vi "Main.vi"() -> ()   [LabVIEW 2020]
uses:
  Main/Main Refs.ctl
  Hardware/Tecan/Pump Config.ctl
  Main/Timing Specs.ctl
  Main/Vacuum Specs.ctl
  Main/Cartridges.ctl
  Main/Cartridge Status.ctl
  Main/Commands.ctl
  Lib/Time/Wells.ctl
  Lib/Time/Bottles.ctl
  Main/Process State.ctl
  Main/Vacuum Test.ctl
  Hardware/Tecan/Pump Control.ctl
  Main/Pump Port.ctl
  Hardware/Tecan/Velocity Units.ctl
  Main/Pump Script Step.ctl
  Main/Script Step.ctl
  Main/Drain Valve.ctl
  Main/Wash Step.ctl
  Main/Zaber Controls.ctl
  Main/Vacuum Output.ctl
  Hardware/DAQ Mngr.ctl
  Main/Process Mngr.ctl
  Main/Cartridge Mngr.ctl
  Main/Script Mngr Action.ctl
  Main/Script Mngr Script choice.ctl
  Main/Time elapsed.ctl
  Hardware/Denkovi Mngr.ctl
  Hardware/Valco Valve/Valco Valve Mngr Action.ctl
  Hardware/Tricon Mngr.ctl
  Hardware/Mot Stage Mngr.ctl
  Main/Config Mngr.ctl
  Hardware/Hardware Globals.vi
  Main/Main Globals.vi
  Lib/Utilities.lvlib
  Hardware/Zaber/Zaber A Series.lvlib
panel:
  in  "Config 2":T1={"Syringe size"=0, "Syringe address"=0, "# of ports"=0, "Init String"="Z0N1R", "Full Stroke (cnts)"=0, "Model"=enum."XC", "TW Position"=0.0, "Load Position"=0.0, "Bottom Position"=0.0, "Station ID"="", "Default Protocol"=path "", "Dry Time(s)"=0.0, "Python Version"="", "NFC SN Array"=["21121521200223", "21121521200186", "21121521200213", "52541737200062"], "Timing"={"Checking pres and leak"=0.0, "Priming input lines"=0.0, "Rinsing syringe"=0.0, "Filling well X w/ X"=0.0, "Drain well X"=0.0, "Clearing wells and lines"=0.0, "Draining wells"=0.0, "Rinsing all wells"=0.0, "Testing for leaks/clogs"=0.0, "Rinsing wells"=0.0}, "Pressure Specs"={"Pressure max"=0.0, "Pressure min"=0.0, "Decay delta"=0.0, "Pressure time"=0.0, "Conf. R"=0.0, "LeakRateMax"=0.0}}
  out "Progress":u8(slide) scale=0.0..100.0
  in  "Software Mode":bool=TRUE
  out "Version":string
  out "error out":errorcluster
  in  "Main References":T4
  in  "Tab Control":T5(tab)
  in  "Init Hardware":bool
  in  "Main Clean Cart":bool
  out "Zaber Found":bool caption="Motion"
  out "Relays Found":bool caption="Relays"
  out "NI DAQ Found":bool caption="DAQ"
  out "Current Protocol":string
  out "Date":string
  out "Station":string="Fixture 1"
  in  "Operator":string
  in  "Time Remaining":string
  in  "Start TW":bool
  in  "Cartridges":T6
  out "Pump Found":bool caption="Pump"
  out "Valco Found":bool caption="Valves"
  in  "Commands":T8={"Drain All Wells"=FALSE, "Rinse All Wells"=FALSE, "Prime"=FALSE, "Well #"=enum."Well 1", "Bottle #"=enum."Bottle 1", "Fill"=FALSE, "Run State"=FALSE, "State"=enum."Fill Wells", "Empty Lines"=FALSE, "Clean&Dry Cartridge"=FALSE, "Check for leaks"=FALSE, "Cart Test Array"=[], "Number of rinses"=0.0} {"Number of rinses" min=1.0 max=50.0 step=1.0}
  in  "Protocol Save":bool
  in  "Protocol Load":bool
  out "Wash Setup File Path":path
  in  "Protocol Clear":bool
  in  "Wash Array":T13[](array[typedef]) {"# of Rinses" max=10}
  in  "Manual Subtab":T14(tab)
  in  "Fit Pnts":dbl
  in  "AutoLock":bool=TRUE
  in  "Zaber Save Bottom Pos":bool
  in  "Zaber Save Load Pos":bool
  in  "Zaber Save TW Pos":bool
  in  "Zaber Bottom_pos":bool
  in  "Zaber Load_pos":bool
  in  "Zaber TW_pos":bool
  in  "Man Cart Read":T15={"Cart1"=TRUE, "Cart2"=TRUE, "Cart3"=TRUE, "Cart4"=TRUE, "Cart 1 SN"="", "Cart 2 SN"="", "Cart 3 SN"="", "Cart 4 SN"=""}
  out "Cart Sense Cluster":T16
  in  "Man Cart Control":T16={"Cart1"=TRUE, "Cart2"=TRUE, "Cart3"=TRUE, "Cart4"=TRUE}
  in  "Man Pres Control":T17={"Vial1"=TRUE, "Vial2"=TRUE, "Vial3"=TRUE, "Vial4"=TRUE, "Vent"=TRUE, "Pressure"=TRUE, "Pinch Valve"=FALSE}
  in  "Man Valco":enum32{"Port1", "Port2", "Port3", "Port4"}(radio)
  in  "Syringe Pump":T18={"Syringe Pos"=0, "Rate"=0.0, "Volume"=0.0, "Valve"=enum."Bottle 1", "Action"=enum."Withdraw", "Move Type"=enum."Rel", "Init"=TRUE, "Empty Syr."=TRUE, "Full Fill"=TRUE, "Units"=enum."ul/s"} {"Syringe Pos" scale=0.0..2500.0}
  in  "Pump Cmd":string
  out "Pump Response":string
  in  "Send Cmd":bool
  in  "Man Peristaltic Ctrl":bool
  out "Pressure Level":cluster{"Time":dbl[], "Value":dbl[]}[](graph)
  in  "Motor Cluster":T21 {"Mot Rel Dist" min=0.0 max=400000.0; "Mot Abs Dist" format="%#.1f"; "Position(mm)" format="%.2f"}
  out "Data Array":T22[](array[typedef])
  in  "Man Script Step":u16
  out "Man Script Path":path
  in  "Man Script Run":bool
  in  "Manual Script Array":T23[](array[typedef])
  in  "Man Script Load":bool
  in  "Man Script Save":bool
  in  "Man Script Clear":bool
  in  "Pump Script Array":T25[](array[typedef])
  in  "Pump Save Script":bool
  in  "Pump Load Script":bool
  in  "Pump Script File":path
  in  "Pump Clear Script":bool
  in  "Pump Start Script":bool
  out "Reports":path
  out "Python Folder":path
  out "Data Folder":path
  out "Root path":path
  out "Config Folder":path
  out "Scripts Folder":path
  out "Logs Folder":path
  in  "Save Config":bool
  in  "Config":T1={"Syringe size"=0, "Syringe address"=0, "# of ports"=0, "Init String"="Z0N1R", "Full Stroke (cnts)"=0, "Model"=enum."XC", "TW Position"=0.0, "Load Position"=0.0, "Bottom Position"=0.0, "Station ID"="", "Default Protocol"=path "", "Dry Time(s)"=0.0, "Python Version"="", "NFC SN Array"=["21121521200223", "21121521200186", "21121521200213", "52541737200062"], "Timing"={"Checking pres and leak"=0.0, "Priming input lines"=0.0, "Rinsing syringe"=0.0, "Filling well X w/ X"=0.0, "Drain well X"=0.0, "Clearing wells and lines"=0.0, "Draining wells"=0.0, "Rinsing all wells"=0.0, "Testing for leaks/clogs"=0.0, "Rinsing wells"=0.0}, "Pressure Specs"={"Pressure max"=0.0, "Pressure min"=0.0, "Decay delta"=0.0, "Pressure time"=0.0, "Conf. R"=0.0, "LeakRateMax"=0.0}}
  out "Protocols Folder":path
  out "Run Time System?":bool
  out "Error":string
  out "Status":string
  # "Tecan Pump"
  # "Pressure"
  # "General"
  # "Timing"
  # "Protocol"
  # "Zaber"
  # "NFC Reader 1"
  # "NFC  Reader 2"
  # "NFC Reader 3"
  # "NFC Reader 4"
  # "Tecan Pump"
  # "Pressure"
  # "General"
  # "Timing"
  # "Protocol"
  # "Zaber"
  # "NFC Reader 1"
  # "NFC  Reader 2"
  # "NFC Reader 3"
  # "NFC Reader 4"
  # "System"
  # "Cartridge Utitlies"
  # "Wells"
  # "times"
  # "from"
  # "State Machine"
  # "System"
  # "Cartridge Utitlies"
  # "Wells"
  # "times"
  # "from"
  # "State Machine"
  # "Wash Protocol"
  # "Tecan Syringe Pump"
  # "Motion"
  # "Cartridges"
  # "Pressure"
  # "Tecan Serial Communication"
  # "Waste"
  # "Step"
  # "Volume"
  # "Rate"
  # "Valco"
  # "Peri"
  # "Pressure"
  # "Move Abs"
  # "Delay(s)"
  # "Tecan Pump"
  # "Pressure"
  # "General"
  # "Timing"
  # "Protocol"
  # "Zaber"
  # "NFC Reader 1"
  # "NFC  Reader 2"
  # "NFC Reader 3"
  # "NFC Reader 4"
  # "Software created by:\nYuri Kouchnir"
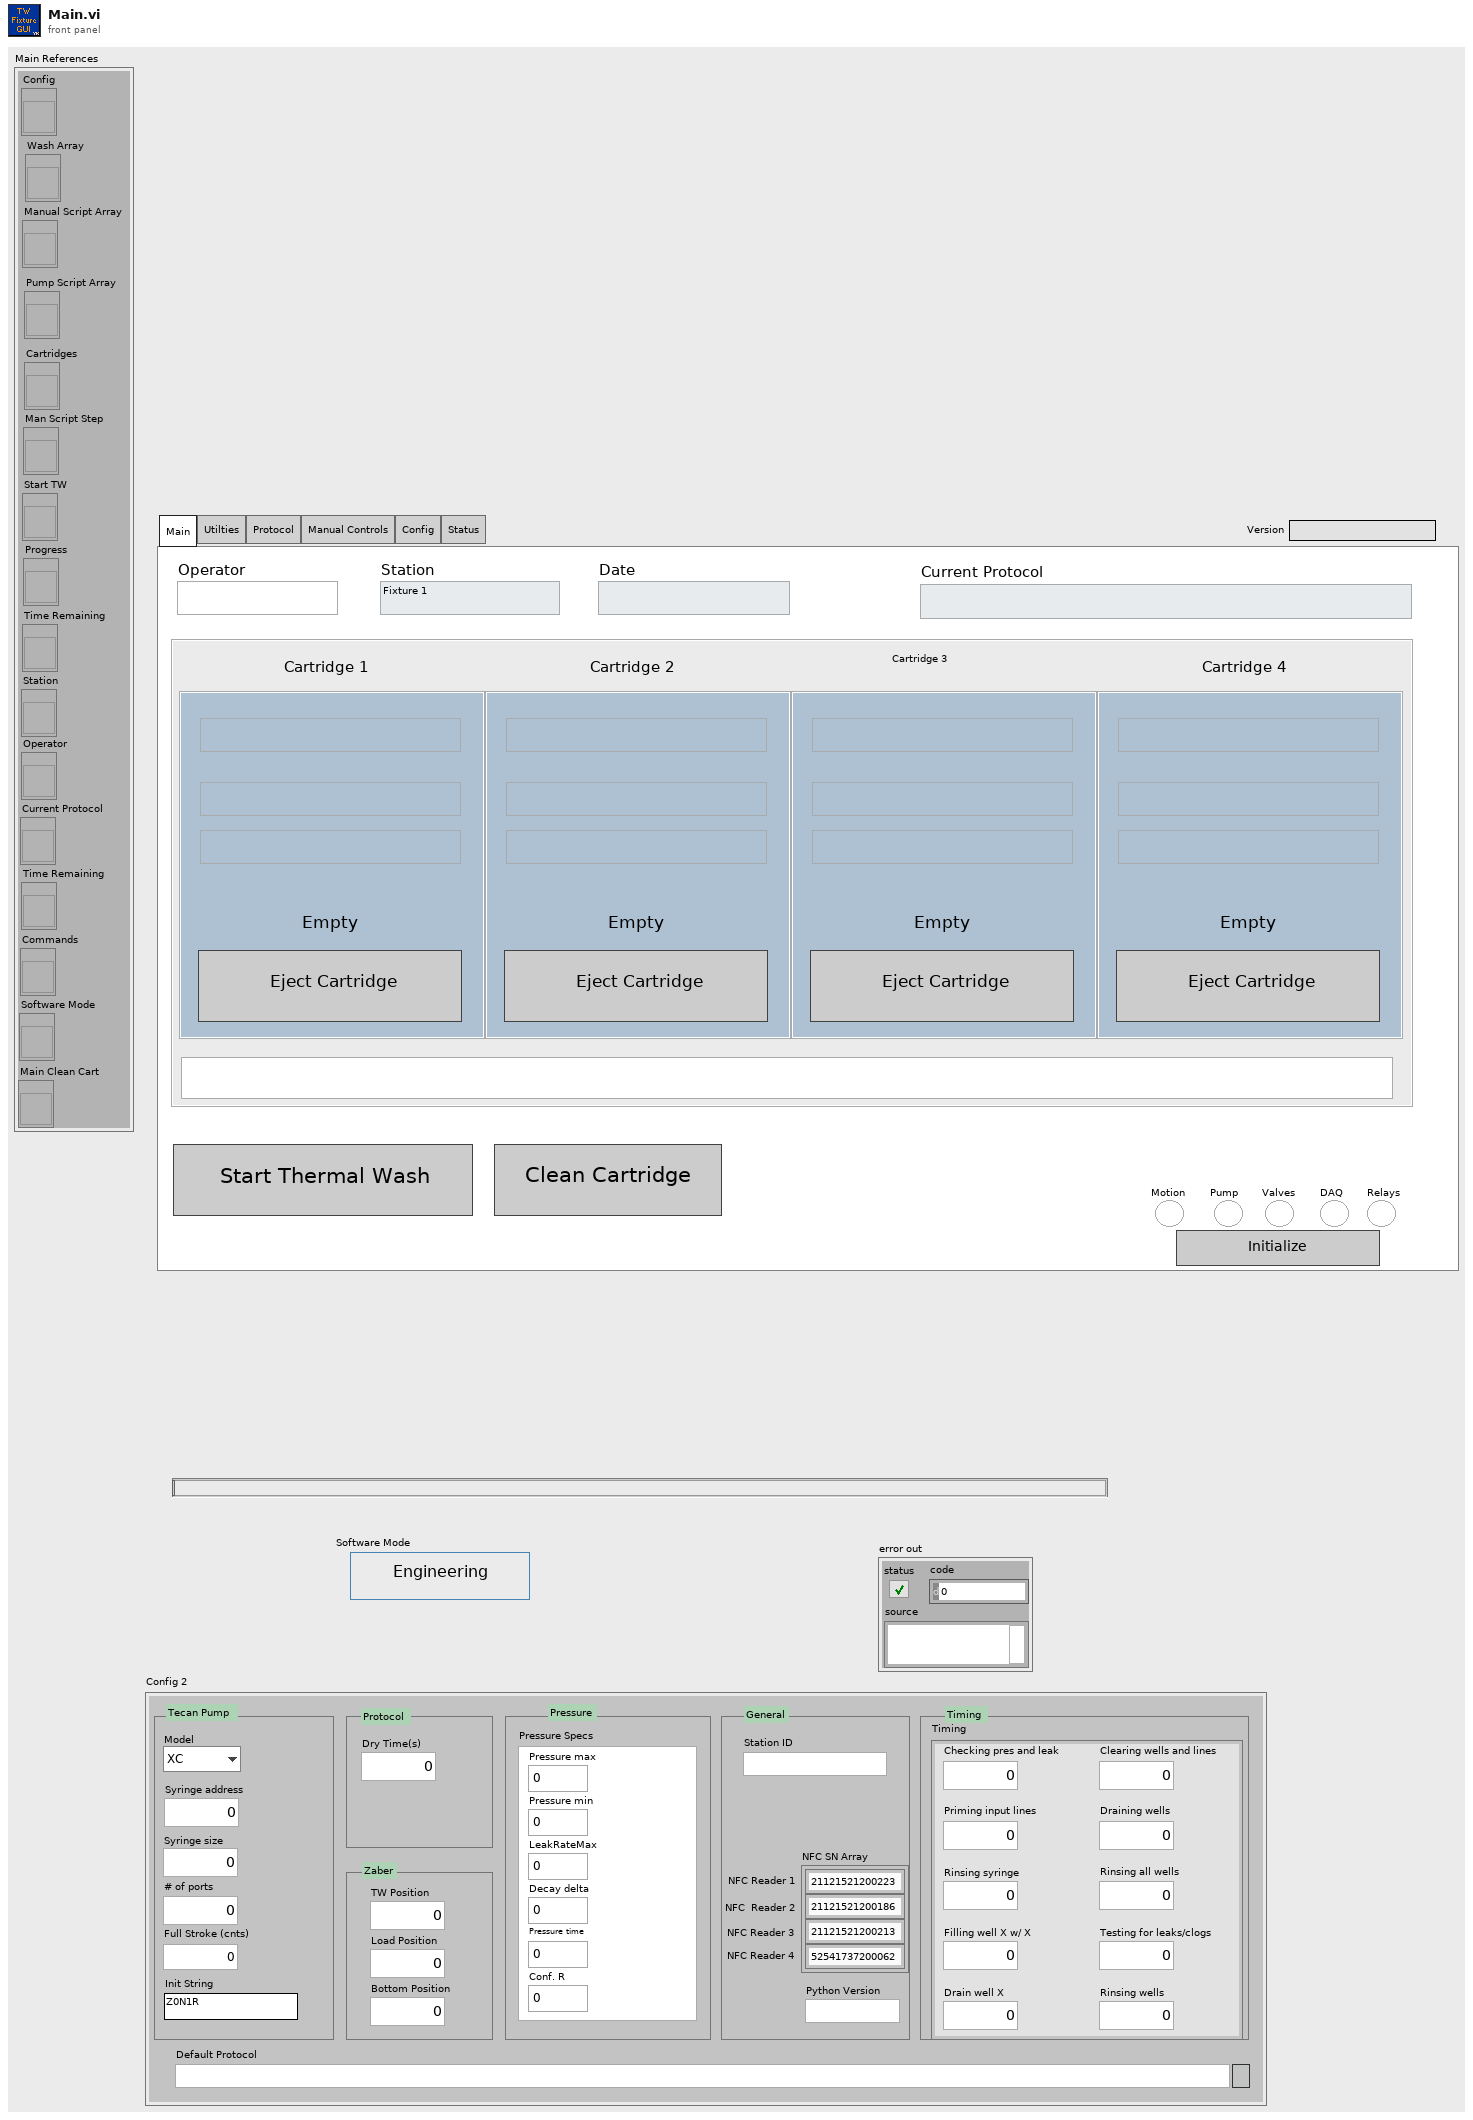
[diagram p1: front panel]
types:
  T1 = typedef "Pump Config.ctl" = cluster{"Syringe size":u32, "Syringe address":u32, "# of ports":u32, "Init String":string, "Full Stroke (cnts)":i32, "Model":enum16{"XC", "Centris"}, "TW Position":dbl, "Load Position":dbl, "Bottom Position":dbl, "Station ID":string, "Default Protocol":path, "Dry Time(s)":dbl, "Python Version":string, "NFC SN Array":string[], "Timing":T2, "Pressure Specs":T3}
  T2 = typedef "Timing Specs.ctl" = cluster{"Checking pres and leak":dbl, "Priming input lines":dbl, "Rinsing syringe":dbl, "Filling well X w/ X":dbl, "Drain well X":dbl, "Clearing wells and lines":dbl, "Draining wells":dbl, "Rinsing all wells":dbl, "Testing for leaks/clogs":dbl, "Rinsing wells":dbl}
  T3 = typedef "Vacuum Specs.ctl" = cluster{"Pressure max":dbl, "Pressure min":dbl, "Decay delta":dbl, "Pressure time":dbl, "Conf. R":dbl, "LeakRateMax":dbl}
  T4 = typedef "Main Refs.ctl" = cluster{"Config":refnum<vi>, "Wash Array":refnum<vi>, "Manual Script Array":refnum<vi>, "Pump Script Array":refnum<vi>, "Cartridges":refnum<vi>, "Man Script Step":refnum<vi>, "Start TW":refnum<vi>, "Progress":refnum<vi>, "Time Remaining":refnum<vi>, "Station":refnum<vi>, "Operator":refnum<vi>, "Current Protocol":refnum<vi>, "Time Remaining":refnum<vi>, "Commands":refnum<vi>, "Software Mode":refnum<vi>, "Main Clean Cart":refnum<vi>}
  T5 = enum32{"Main", "Utilties", "Protocol", "Manual Controls", "Config", "Status"}
  T6 = typedef "Cartridges.ctl" = cluster{"Cartridge 1":T7, "Cartridge 2":T7, "Cartridge 3":T7, "Cartridge 4":T7, "Current Status":string}
  T7 = typedef "Cartridge Status.ctl" = cluster{"Serial Number":string, "Reagent":string, "Cart Status":string, "Inserted":bool, "Eject":bool}
  T8 = typedef "Commands.ctl" = cluster{"Drain All Wells":bool, "Rinse All Wells":bool, "Prime":bool, "Well #":T9, "Bottle #":T10, "Fill":bool, "Run State":bool, "State":T11, "Empty Lines":bool, "Clean&Dry Cartridge":bool, "Check for leaks":bool, "Cart Test Array":T12[], "Number of rinses":dbl}
  T9 = typedef "Wells.ctl" = enum16{"Well 1", "Well 2", "Well 3", "Well 4"}
  T10 = typedef "Bottles.ctl" = enum16{"Bottle 1", "Bottle 2", "Bottle 3", "H2O", "Waste"}
  T11 = typedef "Process State.ctl" = enum16{"Idle", "Init", "Check for SN", "Start TW", "SystemLeakTest", "Prime System", "Rinse Wells", "Fill Wells", "PrePresTest", "Apply Pressure", "PostPresTest", "Drain&Rinse", "Dry", "Report", "Finish", "Abort", "Error", "-rinse wells", "-check cartridge", "-clean cartridge", "-drain all", "-fill well"}
  T12 = typedef "Vacuum Test.ctl" = cluster{"pres after":dbl, "pres before":dbl, "leak liquid":dbl, "leak delta":dbl, "Transition":bool, "Pressure":bool, "R before":bool, "R after":bool, "Reagent":string, "Decay":bool}
  T13 = typedef "Wash Step.ctl" = cluster{"Reagent":string, "Bottle":enum16{"Bottle 1", "Bottle 2", "Bottle 3", "Bottle 4"}, "Wash Time(s)":dbl, "Dwell Time(s)":dbl, "# of Rinses":i16}
  T14 = enum32{"Controls", "State Machine", "Script", "Pump Script"}
  T15 = cluster{"Cart1":bool, "Cart2":bool, "Cart3":bool, "Cart4":bool, "Cart 1 SN":string, "Cart 2 SN":string, "Cart 3 SN":string, "Cart 4 SN":string}
  T16 = cluster{"Cart1":bool, "Cart2":bool, "Cart3":bool, "Cart4":bool}
  T17 = cluster{"Vial1":bool, "Vial2":bool, "Vial3":bool, "Vial4":bool, "Vent":bool, "Pressure":bool, "Pinch Valve":bool}
  T18 = typedef "Pump Control.ctl" = cluster{"Syringe Pos":u32, "Rate":dbl, "Volume":dbl, "Valve":T19, "Action":enum32{"Withdraw", "Dispense", "Stop"}, "Move Type":enum32{"Abs", "Rel"}, "Init":bool, "Empty Syr.":bool, "Full Fill":bool, "Units":T20}
  T19 = typedef "Pump Port.ctl" = enum16{"Bottle 1", "Bottle 2", "Bottle 3", "Bottle 4", "Waste", "Well 1", "Well 2", "Well 3", "Well 4", "Bottle X", "Well X"}
  T20 = typedef "Velocity Units.ctl" = enum16{"ul/s", "ul/min"}
  T21 = typedef "Zaber Controls.ctl" = cluster{"Mot Response":string, "Mot Send Cmd":string, "Mot Home":bool, "Mot Clear Err":bool, "Mot Error":string, "Position(mm)":dbl, "Mot Rel -":bool, "Mot Change Vel":bool, "Mot Max Vel":dbl, "Motor Moving":bool, "Position(cnts)":i64, "Mot Abs Dist":dbl, "Mot Rel Dist":dbl, "Mot Abs Move":bool, "Mot Rel +":bool}
  T22 = typedef "Vacuum Output.ctl" = cluster{"Time(s)":dbl, "Pressure":dbl, "Rate":dbl, "R":dbl}
  T23 = typedef "Script Step.ctl" = cluster{"Step":dbl, "Step En":bool, "Valve":T19, "Syr.Amount":dbl, "Syr.Rate":dbl, "direction":enum32{"withdraw", "dispense"}, "Move Type":enum32{"Abs", "Rel"}, "Pump En":bool, "Drain Valve":T24, "Drain En":bool, "Peristaltic":bool, "Peristaltic En":bool, "Pres1":bool, "Pres2":bool, "Pres3":bool, "Pres4":bool, "Pressure En":bool, "Move Abs":dbl, "Motion En":bool, "Delay(s)":dbl, "Delay En":bool, "Use VacX":bool}
  T24 = typedef "Drain Valve.ctl" = enum16{"Well 1", "Well 2", "Well 3", "Well 4", "Well X"}
  T25 = typedef "Pump Script Step.ctl" = cluster{"Valve":enum16{"Valve 1", "Valve 2", "Valve 3", "Valve 4", "Valve 5", "Valve 6", "Valve 7", "Valve 8", "Valve 9"}, "Syr.Amount":dbl, "Syr.Rate":dbl, "move type":enum32{"rel", "abs"}, "direction":enum32{"withdraw", "dispense"}, "Delay(s)":dbl}
  T26 = enum8{"Enabled", "Disabled", "Disabled and Grayed Out"}
  T27 = enum16{"Init", "Reset", "Read", "Update", "Close"}
  T28 = typedef "Time elapsed.ctl" = enum16{"Start", "Update", "Read"}
  T29 = typedef "Mot Stage Mngr.ctl" = enum16{"Connect", "Init", "Status", "Send Cmd", "Current Pos", "Set Accel", "Set Max Vel", "Home", "Rel Move", "Abs Move", "Close"}
  T30 = typedef "Tricon Mngr.ctl" = enum16{"Init COM", "Set Config", "Init Pump", "Home", "Cmd", "Start Pump", "Set Valve", "Dispense", "Withdraw", "Status", "Close"}
  T31 = typedef "Valco Valve Mngr Action.ctl" = enum16{"Connect", "Init", "Cmd", "Set Valve", "Status", "Close"}
  T32 = typedef "Denkovi Mngr.ctl" = enum16{"Search", "Init", "Set Peristaltic", "Set Pressure", "Pres ON", "Vent&Close", "Set All Relays", "Set One Relay", "Read Relays", "Close"}
  T33 = typedef "Process Mngr.ctl" = enum16{"Init", "Run Step", "Update"}
  T34 = typedef "Cartridge Mngr.ctl" = enum16{"Init", "Update", "Detect", "Lock", "Read SN", "Unlock", "Error"}
  T35 = typedef "Script Mngr Script choice.ctl" = enum16{"Manual Script", "Pump Script", "Wash Setup"}
  T36 = typedef "Script Mngr Action.ctl" = enum16{"Init", "Run Script", "Load Script", "Save Script", "Close"}
  T37 = typedef "Config Mngr.ctl" = enum16{"Init", "Load Config", "Save Config", "Load Protocol", "Save Protocol", "Close"}
  T38 = typedef "DAQ Mngr.ctl" = enum16{"Init", "Read Pressure", "Analyze Pressure", "Read Cartridges", "Lock Cartridge", "Unlock Cartridge", "Read PS", "Pinch Valve Engage", "Pinch Valve Disengage", "Close"}
  T39 = typedef "Pressure Point.ctl" = cluster{"Time":dbl[], "Value":dbl[]}
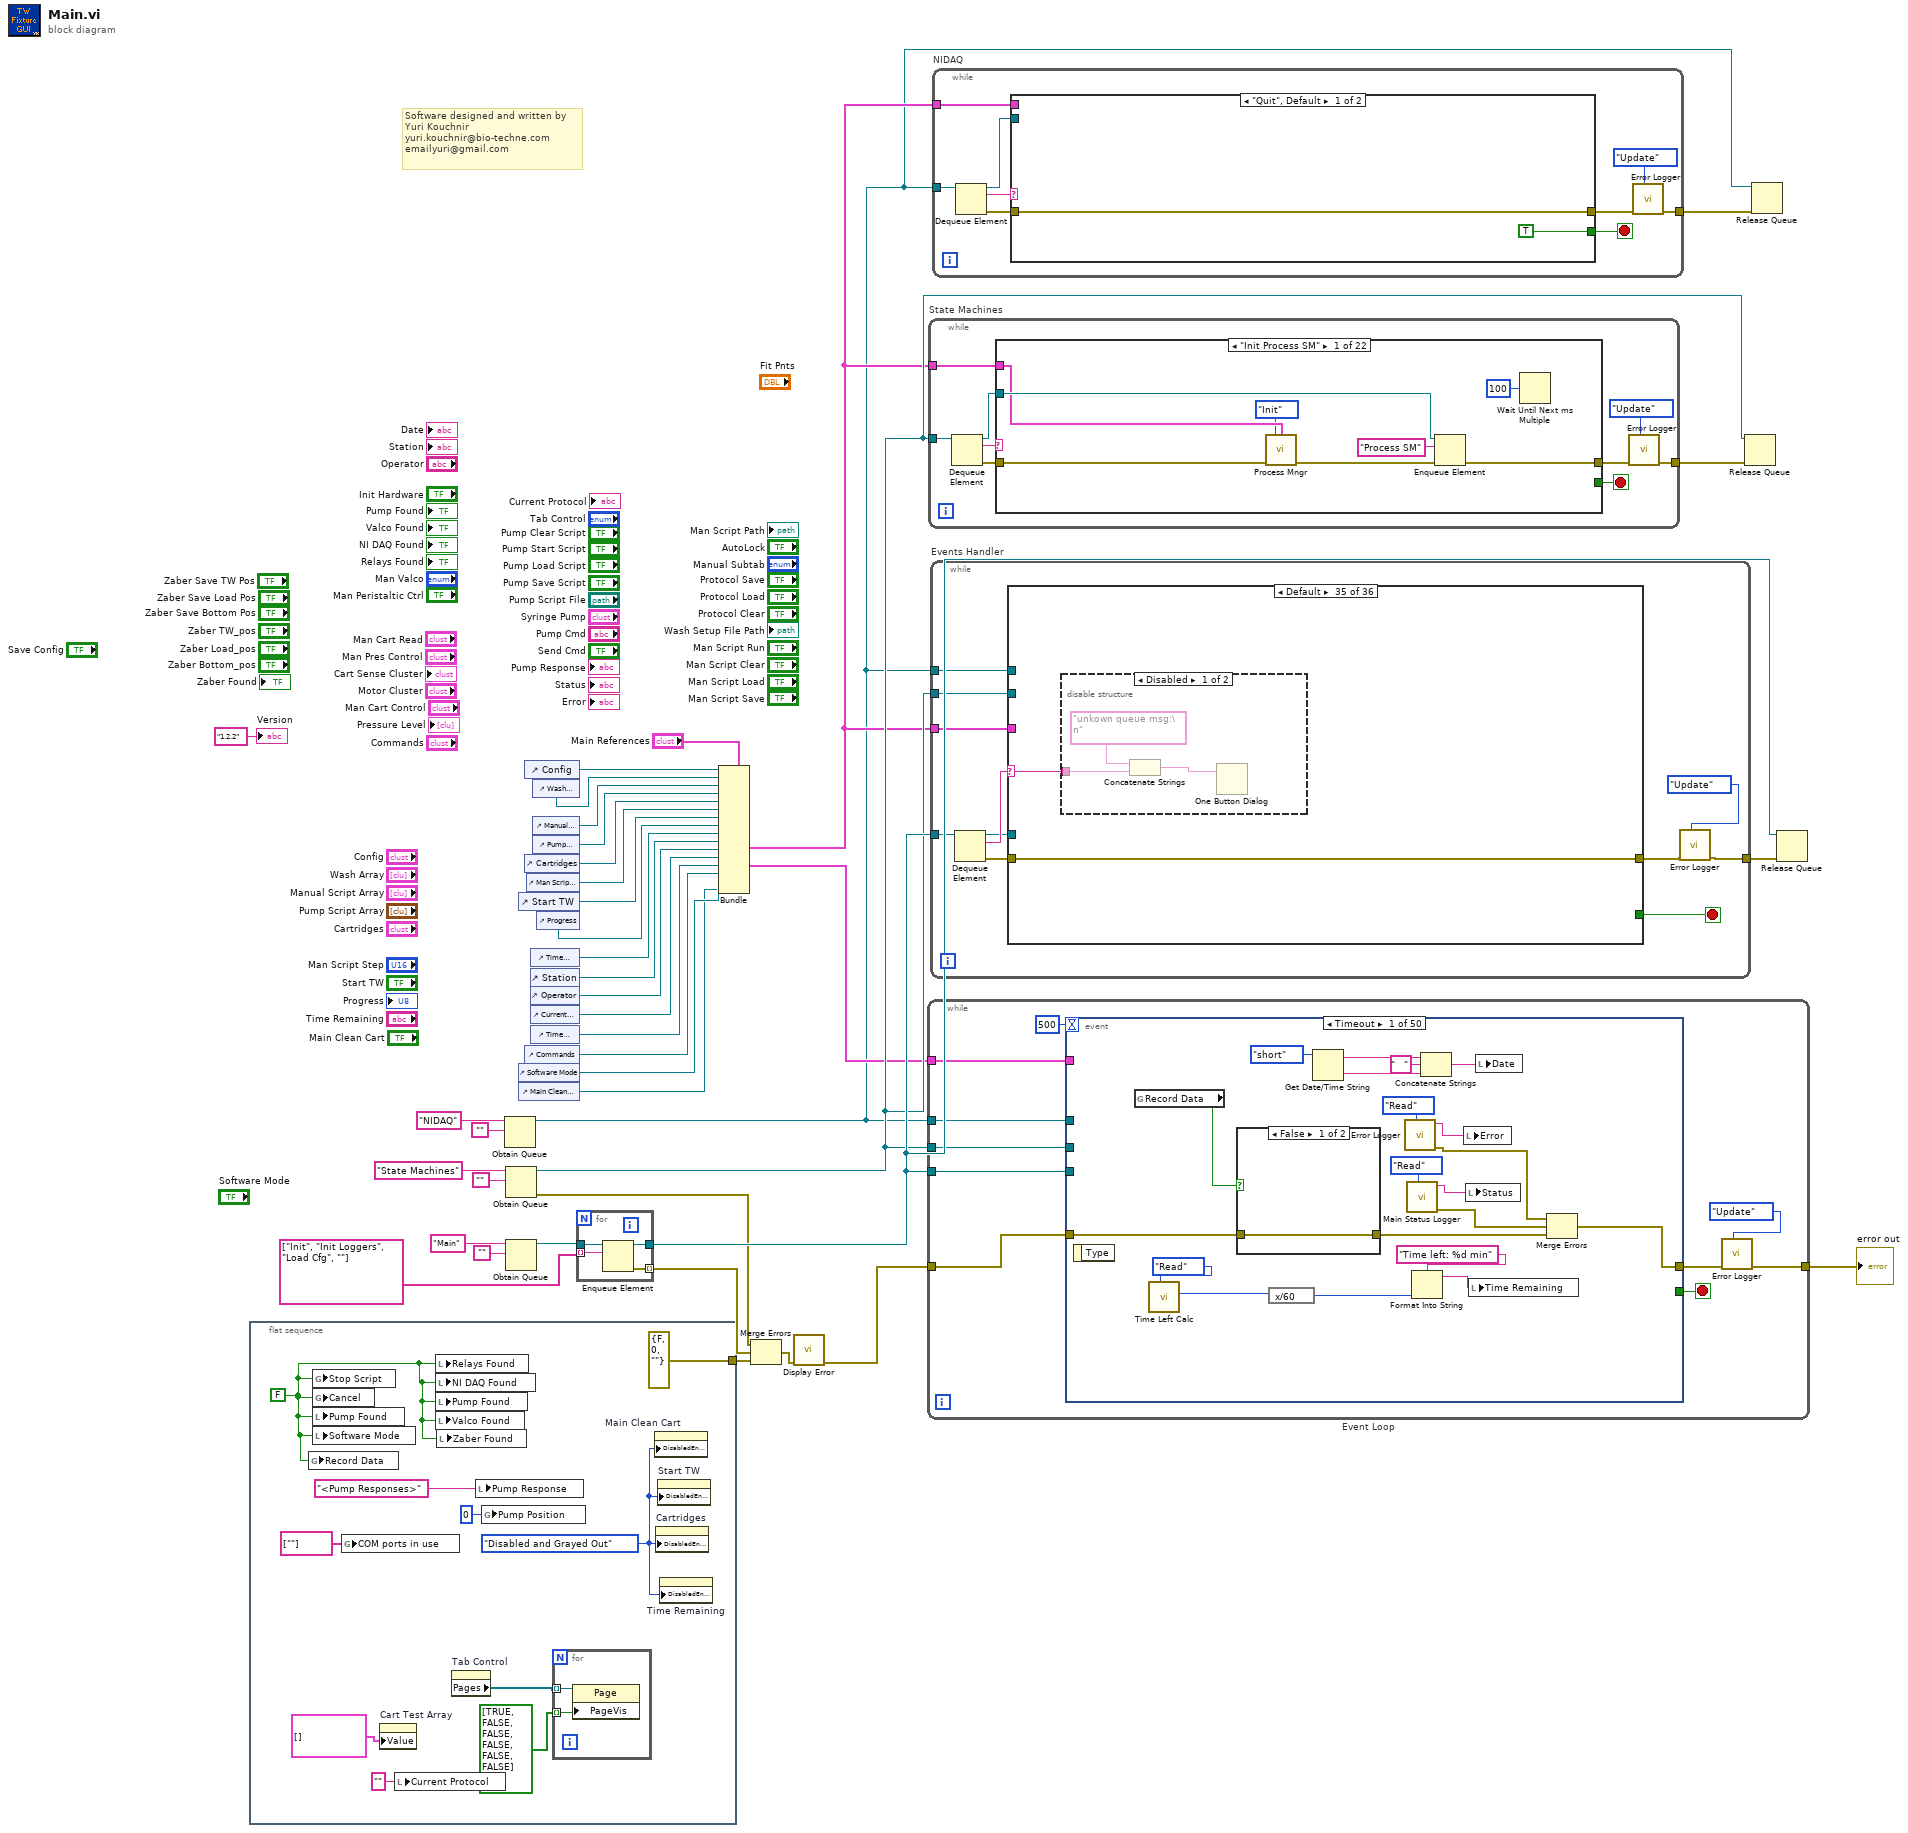
[diagram p0: block diagram]
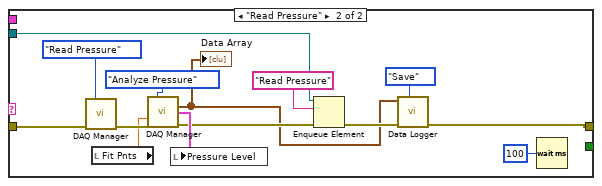
[diagram p2: hidden frame]
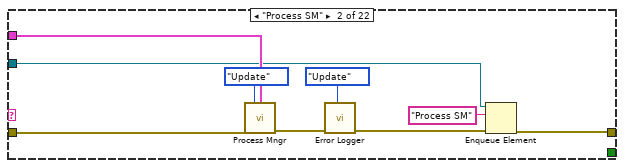
[diagram p3: hidden frame]
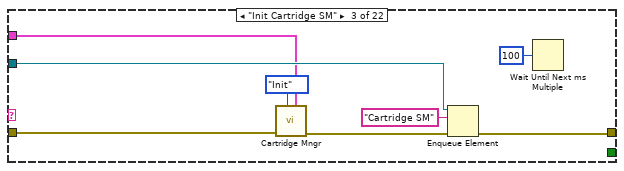
[diagram p4: hidden frame]
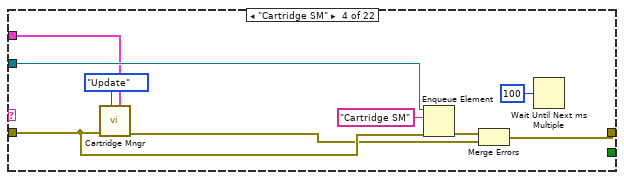
[diagram p5: hidden frame]
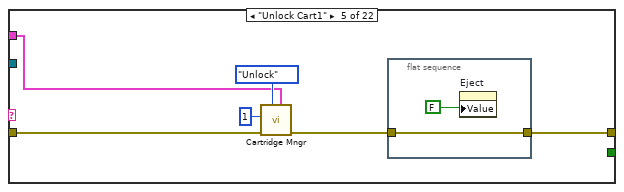
[diagram p6: hidden frame]
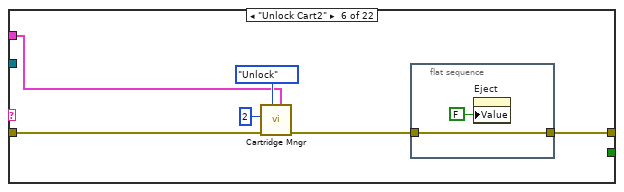
[diagram p7: hidden frame]
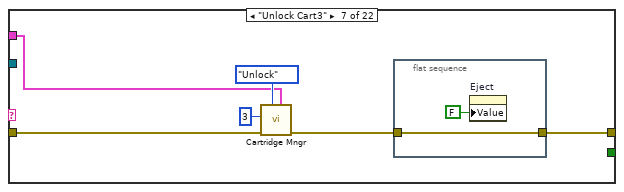
[diagram p8: hidden frame]
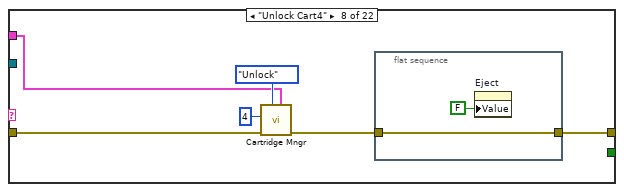
[diagram p9: hidden frame]
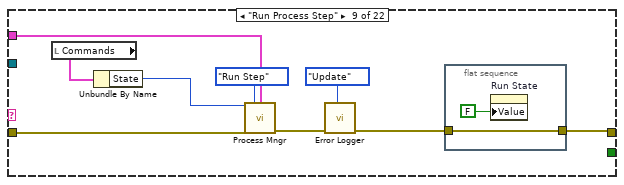
[diagram p10: hidden frame]
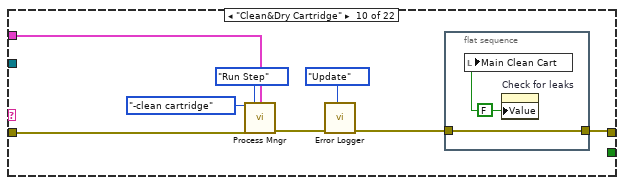
[diagram p11: hidden frame]
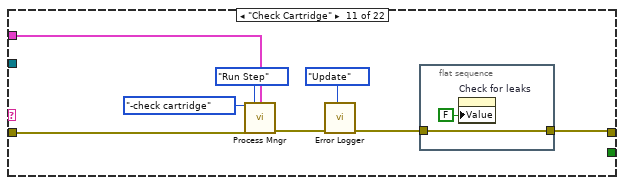
[diagram p12: hidden frame]
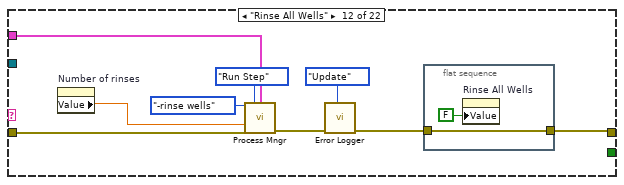
[diagram p13: hidden frame]
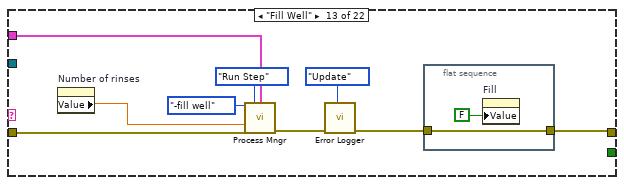
[diagram p14: hidden frame]
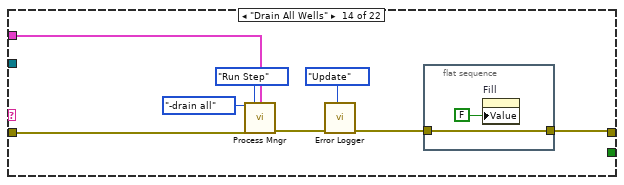
[diagram p15: hidden frame]
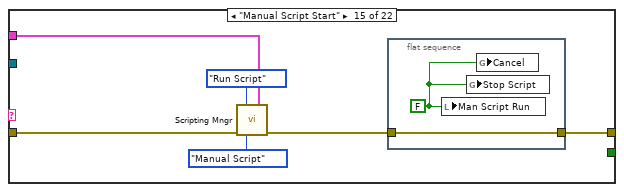
[diagram p16: hidden frame]
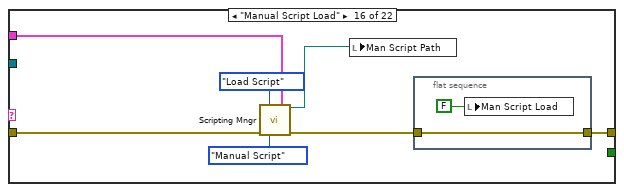
[diagram p17: hidden frame]
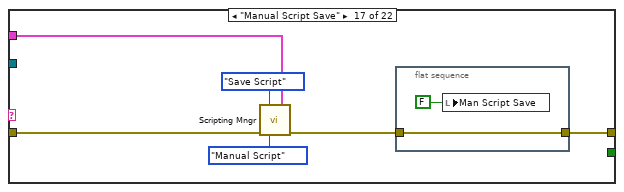
[diagram p18: hidden frame]
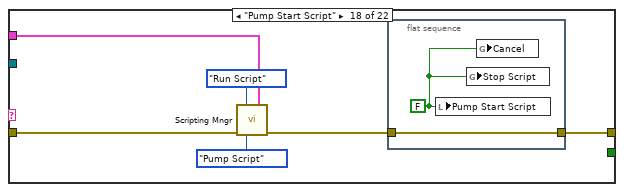
[diagram p19: hidden frame]
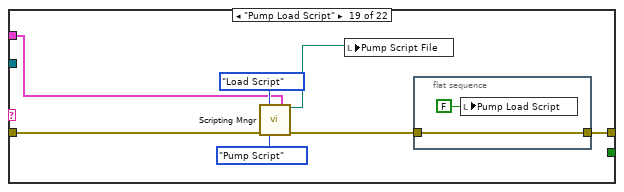
[diagram p20: hidden frame]
diagram:
  # "Software designed and written by\nYuri Kouchnir\nyuri.kouchnir@bio-techne.com\nemailyuri@gmail.com"
  n1 = flat-sequence {
    tunnel: [errorcluster {"status"=FALSE, "code"=0, "source"=""} ("error in (no error)")] -> w34
    frame #0 {
      w40 = T26."Disabled and Grayed Out" ("Disabled")
      w43 = FALSE ("Stop Script")
      n2 = global write "Main Globals.vi" "Record Data"(w43) -> ()
      n3 = global write "Main Globals.vi" "Stop Script"(w43) -> ()
      n4 = global write "Main Globals.vi" "Cancel"(w43) -> ()
      n5 = local write "Pump Found"(w43) -> ()
      n6 = local write "Software Mode"(w43) -> ()
      n7 = global write "Hardware Globals.vi" "COM ports in use"(string[] [""] ("COM ports in use")) -> ()
      n8 = property on="Cart Test Array" class="Arr (strict)"("Value"=T12[] []) -> ()  [unwired: 2 in, 2 out]
      n9 = local write "Current Protocol"("" ("Current Protocol")) -> ()
      n10 = local write "Relays Found"(w43) -> ()
      n11 = local write "NI DAQ Found"(w43) -> ()
      n12 = local write "Pump Found"(w43) -> ()
      n13 = local write "Valco Found"(w43) -> ()
      n14 = local write "Zaber Found"(w43) -> ()
      n15 = property on="Tab Control" class="TabCtl (strict)"() -> ("Pages"=w45:refnum<vi>[])  [unwired: 2 in, 2 out]
      n16 = local write "Pump Response"("<Pump Responses>" ("Pump Response")) -> ()
      n17 = global write "Main Globals.vi" "Pump Position"(u32 0 ("Pump Position")) -> ()
      n18 = for {
        tunnel: w45 -> [w51] mode=indexing
        tunnel: bool[] [TRUE, FALSE, FALSE, FALSE, FALSE, FALSE] -> [w50] mode=indexing
        n19 = property class="Page"(reference=w51, "PageVis"=w50) -> ()  [unwired: 1 in, 2 out]
      }
      n20 = property on="Main Clean Cart" class="Bool (strict)"("DisabledEnum"=w40) -> ()  [unwired: 2 in, 2 out]
      n21 = property on="Cartridges" class="Clust (strict)"("DisabledEnum"=w40) -> ()  [unwired: 2 in, 2 out]
      n22 = property on="Start TW" class="Bool (strict)"("DisabledEnum"=w40) -> ()  [unwired: 2 in, 2 out]
      n23 = property on="Time Remaining" class="Str"("DisabledEnum"=w40) -> ()  [unwired: 2 in, 2 out]
    }
  }
  n24 = Obtain Queue(name (unnamed)="NIDAQ", element data type="") -> (queue out=w8:refnum<queue>)  [unwired: 3 in, 2 out]
  n25 = Obtain Queue(name (unnamed)="State Machines", element data type="") -> (queue out=w21:refnum<queue>, error out=w22:errorcluster)  [unwired: 3 in, 1 out]
  n26 = Obtain Queue(name (unnamed)="Main", element data type="") -> (queue out=w27:refnum<queue>)  [unwired: 3 in, 2 out]
  n27 = control-ref of="Start TW"() -> (w19:refnum<vi>)
  n28 = control-ref of="Software Mode"() -> (w3:refnum<vi>)
  n29 = control-ref of="Main Clean Cart"() -> (w2:refnum<vi>)
  n30 = control-ref of="Config"() -> (w1:refnum<vi>)
  n31 = control-ref of="Cartridges"() -> (w28:refnum<vi>)
  n32 = control-ref of="Commands"() -> (w5:refnum<vi>)
  n33 = control-ref of="Man Script Step"() -> (w18:refnum<vi>)
  n34 = control-ref of="Time Remaining"() -> (w16:refnum<vi>)
  n35 = control-ref of="Station"() -> (w10:refnum<vi>)
  n36 = control-ref of="Operator"() -> (w9:refnum<vi>)
  n37 = control-ref of="Current Protocol"() -> (w4:refnum<vi>)
  n38 = control-ref of="Time Remaining"() -> (w6:refnum<vi>)
  n39 = control-ref of="Wash Array"() -> (w20:refnum<vi>)
  n40 = control-ref of="Manual Script Array"() -> (w7:refnum<vi>)
  n41 = control-ref of="Pump Script Array"() -> (w29:refnum<vi>)
  n42 = control-ref of="Progress"() -> (w17:refnum<vi>)
  n43 = for {
    tunnel: w27 -> [w55]
    tunnel: string[] ["Init", "Init Loggers", "Load Cfg", ""] -> [w54] mode=indexing
    tunnel: [w53] -> w26
    tunnel: [w52] -> w23 mode=indexing
    n44 = Enqueue Element(queue=w55, element=w54) -> (queue out=w53:refnum<queue>, error out=w52:errorcluster)  [unwired: 2 in, 1 out]
  }
  n45 = Bundle(cluster="Main References", "Config"=w1, "Wash Array"=w20, "Manual Script Array"=w7, "Pump Script Array"=w29, "Cartridges"=w28, "Man Script Step"=w18, "Start TW"=w19, "Progress"=w17, "Time Remaining"=w16, "Station"=w10, "Operator"=w9, "Current Protocol"=w4, "Time Remaining"=w6, "Commands"=w5, "Software Mode"=w3, "Main Clean Cart"=w2) -> (w14:T4)
  n46 = Merge Errors(w22, w23, w34) -> (w24:errorcluster)
  n47 = call "Display Error.vi"("error in (no error)"=w24) -> ("error out"=w32:errorcluster)  [unwired: 9 in, 1 out]
  n48 = while "Event Loop" {
    tunnel: w26 -> [w64]
    tunnel: w21 -> [w63]
    tunnel: w32 -> [w61]
    tunnel: w14 -> [w62]
    tunnel: [w56] -> w31
    tunnel: w8 -> [w59]
    stop <- w65 stop-if-true
    n49 = event shown="[0] Timeout" {
      selector: _ -> [_ _ _ _ _ _ _ _ _ _ _ _ _ _ _ _ _ _ _ _ _ _ _ _ _ _ _ _ _ _ _ _ _ _ _ _ _ _ _ _ _ _ _ _ _ _ _ _ _ _]
      dyn-events: _ -> [_ _ _ _ _ _ _ _ _ _ _ _ _ _ _ _ _ _ _ _ _ _ _ _ _ _ _ _ _ _ _ _ _ _ _ _ _ _ _ _ _ _ _ _ _ _ _ _ _ _]
      timeout: 500 -> [_ _ _ _ _ _ _ _ _ _ _ _ _ _ _ _ _ _ _ _ _ _ _ _ _ _ _ _ _ _ _ _ _ _ _ _ _ _ _ _ _ _ _ _ _ _ _ _ _ _]
      tunnel: [_ _ _ TRUE _ _ _ _ _ _ _ _ _ _ _ _ _ _ _ _ _ _ _ _ _ _ _ _ _ _ _ _ _ _ _ _ _ _ _ _ _ _ _ _ _ _ _ _ _ _] -> w65
      tunnel: w64 -> [_ w92 _ w130 _ w145 w155 w157 w159 w161 w163 w165 w167 w169 w171 w173 w175 w177 w179 w181 w183 w185 _ _ _ w199 _ _ _ _ _ _ _ _ _ _ _ _ _ _ _ _ _ _ _ w363 w365 w367 w369 _]
      tunnel: w63 -> [_ _ _ w131 w138 _ _ _ _ _ _ _ _ _ _ _ _ _ _ _ _ _ _ _ _ _ w200 w202 w204 _ w210 _ w232 w250 w270 w287 w303 w319 w338 w347 _ w351 w353 w355 w357 _ _ _ _ _]
      tunnel: w62 -> [_ _ _ _ _ _ _ _ _ _ _ _ _ _ _ _ _ _ _ _ _ _ _ _ _ _ _ _ _ _ _ w220 w233 w251 w271 w288 w304 w320 _ _ _ _ _ _ _ _ _ _ _ _]
      tunnel: w61 -> [w84 _ _ w127 _ _ _ _ _ _ _ _ _ _ _ _ _ _ _ _ _ _ _ _ _ _ _ _ _ _ _ _ _ _ _ _ _ _ _ _ _ _ _ _ _ _ _ _ _ _]
      tunnel: [w78 w93 w111 w125 _ _ _ _ _ _ _ _ _ _ _ _ _ _ _ _ _ _ _ _ _ _ _ _ _ _ _ w219 w234 w252 w272 w289 w305 w321 _ _ _ _ _ _ _ _ _ _ _ _] -> w57
      tunnel: w59 -> [_ _ _ w128 _ _ _ _ _ _ _ _ _ _ _ _ _ _ _ _ _ _ _ _ _ _ _ _ _ _ _ _ _ _ _ _ _ _ _ _ _ _ _ _ _ _ _ _ _ _]
      event Timeout {
        n50 = event-data() -> ()  [unwired: 1 in, 1 out]
        n51 = global read "Main Globals.vi" "Record Data"() -> (w85:bool)
        n52 = call "Time Left Calc.vi"("Enum"=Time_elapsed."Read") -> ("Time Left"=w67:u32)  [unwired: 8 in, 2 out]
        n53 = case shown="False" w85 {
          tunnel: w84 -> [w86 w88]
          tunnel: [w86 w87] -> w79
          frame False {
          }
          frame True {
            n54 = global read "Main Globals.vi" "data file path"() -> (w89:path)
            n55 = call "Write Data.vi"("error in (no error)"=w88, "file (use dialog)"=w89) -> ("error out"=w87:errorcluster)  [unwired: 9 in]
          }
        }
        n56 = expression code="x/60"(w67) -> (w66:u32)
        n57 = Get Date/Time String(date format (0)=enum16{"short", "long", "abbreviated"}."short") -> (date string=w74:string, time string=w73:string)  [unwired: 2 in]
        n58 = call "Error Logger.vi"("Action"=T27."Read") -> ("error out"=w76:errorcluster, "Log"=w81:string)  [unwired: 9 in]
        n59 = call "Main Status Logger.vi"("Action"=T27."Read") -> ("error out"=w77:errorcluster, "Log"=w80:string)  [unwired: 9 in]
        n60 = Format Into String(format string="Time left: %d min", w66) -> (resulting string=w68:string)  [unwired: 2 in, 1 out]
        n61 = Concatenate Strings(w74, "   " ("string"), w73) -> (w71:string)
        n62 = local write "Error"(w81) -> ()
        n63 = local write "Status"(w80) -> ()
        n64 = local write "Time Remaining"(w68) -> ()
        n65 = local write "Date"(w71) -> ()
        n66 = Merge Errors(w76, w77, w79) -> (w78:errorcluster)
      }
      event "Init Hardware": Mouse Up {
        n67 = event-data() -> ()  [unwired: 1 in, 4 out]
        n68 = flat-sequence {
          tunnel: [w99] -> w94
          tunnel: w92 -> [w97]
          tunnel: [w97] -> w91
          tunnel: [w95] -> w90
          tunnel: w94 -> [w109]
          tunnel: [w109] -> w93
          tunnel: w91 -> [w108]
          tunnel: w90 -> [_]
          frame #0 {
            w95 = T26."Disabled and Grayed Out" ("Disabled")
            w98 = FALSE ("Zaber Found")
            n69 = local write "Zaber Found"(w98) -> ()
            n70 = local write "Relays Found"(w98) -> ()
            n71 = local write "Pump Found"(w98) -> ()
            n72 = local write "Valco Found"(w98) -> ()
            n73 = local write "NI DAQ Found"(w98) -> ()
            n74 = global write "Hardware Globals.vi" "COM ports in use"(string[] [] ("COM ports in use")) -> ()
            n75 = property on="Main Clean Cart" class="Bool (strict)"("DisabledEnum"=w95) -> ()  [unwired: 2 in, 2 out]
            n76 = call "Denkovi Manager.vi"("Action"=Denkovi_Mngr."Close") -> ("error out"=w105:errorcluster)  [unwired: 8 in, 2 out]
            n77 = property on="Start TW" class="Bool (strict)"("DisabledEnum"=w95) -> ()  [unwired: 2 in, 2 out]
            n78 = call "Valco Valve Mngr.vi"("Mngr Action"=Valco_Valve_Mngr_Action."Close", "error in (no error)"=w105) -> ("error out"=w102:errorcluster)  [unwired: 9 in, 4 out]
            n79 = property on="Cartridges" class="Clust (strict)"("DisabledEnum"=w95) -> ()  [unwired: 2 in, 2 out]
            n80 = call "Tecan Mngr.vi"("Address"=u8 1, "Mngr Action"=Tricon_Mngr."Close", "error in (no error)"=w102) -> ("error out"=w100:errorcluster)  [unwired: 7 in, 5 out]
            n81 = call "Zaber Manager.vi"("Action"=Mot_Stage_Mngr."Close", "error in (no error)"=w100) -> ("error out"=w99:errorcluster)  [unwired: 7 in, 6 out]
          }
          frame #1 {
            n82 = Enqueue Element(queue=w108, element="Init Hardware") -> ()  [unwired: 2 in, 3 out]
          }
        }
      }
      event "Software Mode": Value Change {
        n83 = event-data() -> ("NewVal"=w112:bool)  [unwired: 1 in]
        n84 = case shown="True" w112 {
          tunnel: [w113 _] -> w111
          frame True {
            n85 = call "Password Popup.vi"() -> ("error out"=w113:errorcluster, "Password out"=w114:string)  [unwired: 10 in]
            n86 = Equal?(x="firefly", y=w114) -> (x = y?=w115:bool)
            n87 = case shown="True" w115 {
              frame False {
              }
              frame True {
                n88 = property on="Tab Control" class="TabCtl (strict)"() -> ("Pages"=w117:refnum<vi>[])  [unwired: 2 in, 2 out]
                n89 = for {
                  tunnel: w117 -> [w120] mode=indexing
                  tunnel: bool[] [TRUE, TRUE, TRUE, TRUE, TRUE, TRUE] -> [w119] mode=indexing
                  n90 = property class="Page"(reference=w120, "PageVis"=w119) -> ()  [unwired: 1 in, 2 out]
                }
              }
            }
          }
          frame False {
            n91 = property on="Tab Control" class="TabCtl (strict)"() -> ("Pages"=w121:refnum<vi>[])  [unwired: 2 in, 2 out]
            n92 = for {
              tunnel: w121 -> [w124] mode=indexing
              tunnel: bool[] [TRUE, FALSE, FALSE, FALSE, FALSE, FALSE] -> [w123] mode=indexing
              n93 = property class="Page"(reference=w124, "PageVis"=w123) -> ()  [unwired: 1 in, 2 out]
            }
          }
        }
      }
      event Panel Close? {
        n94 = event-data() -> ()  [unwired: 1 in, 1 out]
        n95 = Build Array(w128, w131, w130) -> (w129:refnum<queue>[])
        n96 = for {
          tunnel: w129 -> [w136] mode=indexing
          tunnel: w127 -> [w135]
          tunnel: [w134] -> w126 mode=indexing
          n97 = Enqueue Element At Opposite End(queue=w136, element="Quit", error in (no error)=w135) -> (error out=w134:errorcluster)  [unwired: 1 in, 2 out]
        }
        n98 = Merge Errors(w126) -> (w125:errorcluster)
        n99 = event-data("Discard?"=TRUE) -> ()  [unwired: 1 in, 1 out]
      }
      event "AutoLock": Value Change {
        n100 = event-data() -> ("NewVal"=w139:bool)  [unwired: 1 in, 5 out]
        n101 = case shown="True" w139 {
          tunnel: w138 -> [_ w141]
          frame False {
          }
          frame True {
            n102 = Enqueue Element(queue=w141, element="Init Cartridge SM") -> ()  [unwired: 2 in, 3 out]
          }
        }
      }
      event Value Change {
        n103 = event-data() -> ("NewVal"=w144:enum32{"Withdraw", "Dispense", "Stop"})  [unwired: 1 in]
        n104 = flat-sequence {
          tunnel: w144 -> [w147]
          tunnel: w145 -> [w148]
          tunnel: [w148] -> w143
          tunnel: [w147] -> w142
          tunnel: w143 -> [w150]
          tunnel: w142 -> [w149]
          frame #0 {
            n105 = global write "Main Globals.vi" "Cancel"(FALSE ("Cancel")) -> ()
          }
          frame #1 {
            n106 = case shown="\"Withdraw\", \"Dispense\"" w149 {
              tunnel: w150 -> [_ w153]
              frame "Stop" {
                n107 = global write "Main Globals.vi" "Cancel"(TRUE ("Cancel")) -> ()
              }
              frame "Withdraw", "Dispense" {
                n108 = Enqueue Element(queue=w153, element="Pump Start") -> ()  [unwired: 2 in, 3 out]
              }
            }
          }
        }
      }
      event Value Change {
        n109 = event-data() -> ()  [unwired: 1 in, 1 out]
        n110 = Enqueue Element(queue=w155, element="Pump Set Valve") -> ()  [unwired: 2 in, 3 out]
      }
      event "Man Pres Control": Value Change {
        n111 = event-data() -> ()  [unwired: 1 in, 1 out]
        n112 = Enqueue Element(queue=w157, element="Relay Pressure") -> ()  [unwired: 2 in, 3 out]
      }
      event "Man Peristaltic Ctrl": Value Change {
        n113 = event-data() -> ()  [unwired: 1 in, 1 out]
        n114 = Enqueue Element(queue=w159, element="Relay Peristaltic") -> ()  [unwired: 2 in, 3 out]
      }
      event "Man Valco": Value Change {
        n115 = event-data() -> ()  [unwired: 1 in, 1 out]
        n116 = Enqueue Element(queue=w161, element="Valco Set") -> ()  [unwired: 2 in, 3 out]
      }
      event "Man Cart Control.Cart1": Value Change {
        n117 = event-data() -> ()  [unwired: 1 in, 1 out]
        n118 = Enqueue Element(queue=w163, element="DAQ Toggle Cart1") -> ()  [unwired: 2 in, 3 out]
      }
      event "Man Cart Control.Cart2": Value Change {
        n119 = event-data() -> ()  [unwired: 1 in, 1 out]
        n120 = Enqueue Element(queue=w165, element="DAQ Toggle Cart2") -> ()  [unwired: 2 in, 3 out]
      }
      event "Man Cart Control.Cart3": Value Change {
        n121 = event-data() -> ()  [unwired: 1 in, 1 out]
        n122 = Enqueue Element(queue=w167, element="DAQ Toggle Cart3") -> ()  [unwired: 2 in, 3 out]
      }
      event "Man Cart Control.Cart4": Value Change {
        n123 = event-data() -> ()  [unwired: 1 in, 1 out]
        n124 = Enqueue Element(queue=w169, element="DAQ Toggle Cart4") -> ()  [unwired: 2 in, 3 out]
      }
      event Value Change {
        n125 = event-data() -> ()  [unwired: 1 in, 1 out]
        n126 = Enqueue Element(queue=w171, element="Zaber Abs Move") -> ()  [unwired: 2 in, 3 out]
      }
      event Value Change {
        n127 = event-data() -> ()  [unwired: 1 in, 1 out]
        n128 = Enqueue Element(queue=w173, element="Zaber Rel Move-") -> ()  [unwired: 2 in, 3 out]
      }
      event Value Change {
        n129 = event-data() -> ()  [unwired: 1 in, 1 out]
        n130 = Enqueue Element(queue=w175, element="Zaber Rel Move+") -> ()  [unwired: 2 in, 3 out]
      }
      event Value Change {
        n131 = event-data() -> ()  [unwired: 1 in, 1 out]
        n132 = Enqueue Element(queue=w177, element="Zaber Home") -> ()  [unwired: 2 in, 3 out]
      }
      event Value Change {
        n133 = event-data() -> ()  [unwired: 1 in, 1 out]
        n134 = Enqueue Element(queue=w179, element="Zaber Set Vel") -> ()  [unwired: 2 in, 3 out]
      }
      event "Zaber TW_pos": Value Change {
        n135 = event-data() -> ()  [unwired: 1 in, 1 out]
        n136 = Enqueue Element(queue=w181, element="Zaber TW_pos") -> ()  [unwired: 2 in, 3 out]
      }
      event "Zaber Load_pos": Value Change {
        n137 = event-data() -> ()  [unwired: 1 in, 1 out]
        n138 = Enqueue Element(queue=w183, element="Zaber Load_pos") -> ()  [unwired: 2 in, 3 out]
      }
      event "Zaber Bottom_pos": Value Change {
        n139 = event-data() -> ()  [unwired: 1 in, 1 out]
        n140 = Enqueue Element(queue=w185, element="Zaber Bottom_pos") -> ()  [unwired: 2 in, 3 out]
      }
      event "Zaber Save TW Pos": Value Change {
        n141 = event-data() -> ()  [unwired: 1 in, 1 out]
        n142 = local read "Motor Cluster"() -> (w189:T21)
        n143 = Unbundle By Name(w189) -> ("Position(mm)"=w187:dbl)
        n144 = local read "Config"() -> (w188:T1)
        n145 = Bundle By Name(cluster=w188, "TW Position"=w187) -> (w186:T1)
        n146 = local write "Config"(w186) -> ()
      }
      event "Zaber Save Load Pos": Value Change {
        n147 = event-data() -> ()  [unwired: 1 in, 1 out]
        n148 = local read "Motor Cluster"() -> (w193:T21)
        n149 = Unbundle By Name(w193) -> ("Position(mm)"=w191:dbl)
        n150 = local read "Config"() -> (w192:T1)
        n151 = Bundle By Name(cluster=w192, "Load Position"=w191) -> (w190:T1)
        n152 = local write "Config"(w190) -> ()
      }
      event "Zaber Save Bottom Pos": Value Change {
        n153 = event-data() -> ()  [unwired: 1 in, 1 out]
        n154 = local read "Motor Cluster"() -> (w197:T21)
        n155 = Unbundle By Name(w197) -> ("Position(mm)"=w195:dbl)
        n156 = local read "Config"() -> (w196:T1)
        n157 = Bundle By Name(cluster=w196, "Bottom Position"=w195) -> (w194:T1)
        n158 = local write "Config"(w194) -> ()
      }
      event "Send Cmd": Value Change {
        n159 = event-data() -> ()  [unwired: 1 in, 1 out]
        n160 = Enqueue Element(queue=w199, element="Pump - Send Cmd") -> ()  [unwired: 2 in, 3 out]
      }
      event "Pump Save Script": Value Change {
        n161 = event-data() -> ()  [unwired: 1 in, 1 out]
        n162 = Enqueue Element(queue=w200, element="Pump Save Script") -> ()  [unwired: 2 in, 3 out]
      }
      event "Man Script Save": Value Change {
        n163 = event-data() -> ()  [unwired: 1 in, 1 out]
        n164 = Enqueue Element(queue=w202, element="Manual Script Save") -> ()  [unwired: 2 in, 3 out]
      }
      event "Man Script Load": Value Change {
        n165 = event-data() -> ()  [unwired: 1 in, 1 out]
        n166 = Enqueue Element(queue=w204, element="Manual Script Load") -> ()  [unwired: 2 in, 3 out]
      }
      event "Man Script Clear": Value Change {
        n167 = event-data() -> ()  [unwired: 1 in, 1 out]
        n168 = local write "Manual Script Array"(T23[] [] ("Manual Script Array")) -> ()
      }
      event "Pump Start Script": Value Change {
        n169 = event-data() -> ("NewVal"=w209:bool)  [unwired: 1 in]
        n170 = flat-sequence {
          tunnel: w209 -> [w212]
          tunnel: w210 -> [w213]
          tunnel: [w213] -> w208
          tunnel: [w212] -> w207
          tunnel: w208 -> [w215]
          tunnel: w207 -> [w214]
          frame #0 {
            n171 = global write "Main Globals.vi" "Cancel"(FALSE ("Cancel")) -> ()
          }
          frame #1 {
            n172 = case shown="True" w214 {
              tunnel: w215 -> [_ w217]
              frame False {
                n173 = global write "Main Globals.vi" "Cancel"(TRUE ("Cancel")) -> ()
              }
              frame True {
                n174 = Enqueue Element(queue=w217, element="Pump Start Script") -> ()  [unwired: 2 in, 3 out]
              }
            }
          }
        }
      }
      event "Start TW": Value Change {
        n175 = event-data() -> ("NewVal"=w221:bool)  [unwired: 1 in, 5 out]
        n176 = case shown="False" w221 {
          tunnel: w220 -> [w223 _]
          tunnel: [w222 _] -> w219
          frame False {
            n177 = flat-sequence {
              tunnel: w223 -> [w230]
              tunnel: [w227] -> w222
              frame #0 {
                n178 = global write "Main Globals.vi" "Cancel"(TRUE ("Cancel")) -> ()
              }
              frame #1 {
                n179 = global read "Hardware Globals.vi" "Zaber VISA"() -> (w229:refnum<visa-resource-name>)
                n180 = call "Stop.vi"("VISA resource name"=w229) -> ("error out"=w228:errorcluster)  [unwired: 9 in, 1 out]
                n181 = call "Process Mngr.vi"("State In"=Process_State."Abort", "Mngr Action"=Process_Mngr."Run Step", "FP"=w230, "error in (no error)"=w228, "Config"="Config 2") -> ("error out"=w227:errorcluster)  [unwired: 9 in, 1 out]
              }
            }
          }
          frame True {
          }
        }
      }
      event Value Change {
        n182 = event-data() -> ("NewVal"=w237:bool)  [unwired: 1 in]
        n183 = local read "Commands"() -> (w236:T8)
        n184 = Unbundle By Name(w236) -> ("State"=w235:T11)
        n185 = case shown="True" w237 {
          tunnel: w235 -> [_ _]
          tunnel: w233 -> [_ _]
          tunnel: [w239 w247] -> w234
          tunnel: w233 -> [w238 _]
          tunnel: w232 -> [_ w249]
          frame False {
            n186 = flat-sequence {
              tunnel: w238 -> [w245]
              tunnel: [w242] -> w239
              frame #0 {
                n187 = global write "Main Globals.vi" "Cancel"(TRUE ("Cancel")) -> ()
              }
              frame #1 {
                n188 = global read "Hardware Globals.vi" "Zaber VISA"() -> (w244:refnum<visa-resource-name>)
                n189 = call "Stop.vi"("VISA resource name"=w244) -> ("error out"=w243:errorcluster)  [unwired: 9 in, 1 out]
                n190 = call "Process Mngr.vi"("State In"=Process_State."Abort", "Mngr Action"=Process_Mngr."Run Step", "FP"=w245, "error in (no error)"=w243) -> ("error out"=w242:errorcluster)  [unwired: 10 in, 1 out]
              }
            }
          }
          frame True {
            n191 = Enqueue Element(queue=w249, element="Run Process Step") -> (error out=w247:errorcluster)  [unwired: 2 in, 2 out]
          }
        }
      }
      event "Main Clean Cart": Value Change {
        n192 = event-data() -> ("NewVal"=w255:bool)  [unwired: 1 in]
        n193 = local read "Commands"() -> (w254:T8)
        n194 = Unbundle By Name(w254) -> ("State"=w253:T11)
        n195 = case shown="False" w255 {
          tunnel: w253 -> [_ _]
          tunnel: w251 -> [_ _]
          tunnel: [w257 w267] -> w252
          tunnel: w251 -> [w256 _]
          tunnel: w250 -> [_ w269]
          frame False {
            n196 = flat-sequence {
              tunnel: w256 -> [w264]
              tunnel: [w261] -> w257
              frame #0 {
                w258 = FALSE ("Main Clean Cart")
                n197 = local write "Main Clean Cart"(w258) -> ()
                n198 = property on="Clean&Dry Cartridge" class="Bool (strict)"("Value"=w258) -> ()  [unwired: 2 in, 2 out]
                n199 = global write "Main Globals.vi" "Cancel"(TRUE ("Cancel")) -> ()
              }
              frame #1 {
                n200 = global read "Hardware Globals.vi" "Zaber VISA"() -> (w263:refnum<visa-resource-name>)
                n201 = call "Stop.vi"("VISA resource name"=w263) -> ("error out"=w262:errorcluster)  [unwired: 9 in, 1 out]
                n202 = call "Process Mngr.vi"("State In"=Process_State."Abort", "Mngr Action"=Process_Mngr."Run Step", "FP"=w264, "error in (no error)"=w262) -> ("error out"=w261:errorcluster)  [unwired: 10 in, 1 out]
              }
            }
          }
          frame True {
            w266 = TRUE ("Main Clean Cart")
            n203 = Enqueue Element(queue=w269, element="Clean&Dry Cartridge") -> (error out=w267:errorcluster)  [unwired: 2 in, 2 out]
            n204 = local write "Main Clean Cart"(w266) -> ()
            n205 = property on="Clean&Dry Cartridge" class="Bool (strict)"("Value"=w266) -> ()  [unwired: 2 in, 2 out]
          }
        }
      }
      event Value Change {
        n206 = event-data() -> ("NewVal"=w273:bool)  [unwired: 1 in]
        n207 = case shown="True" w273 {
          tunnel: w271 -> [_ _]
          tunnel: [w275 w284] -> w272
          tunnel: w271 -> [w274 _]
          tunnel: w270 -> [_ w286]
          frame False {
            n208 = flat-sequence {
              tunnel: w274 -> [w281]
              tunnel: [w278] -> w275
              frame #0 {
                n209 = global write "Main Globals.vi" "Cancel"(TRUE ("Cancel")) -> ()
              }
              frame #1 {
                n210 = global read "Hardware Globals.vi" "Zaber VISA"() -> (w280:refnum<visa-resource-name>)
                n211 = call "Stop.vi"("VISA resource name"=w280) -> ("error out"=w279:errorcluster)  [unwired: 9 in, 1 out]
                n212 = call "Process Mngr.vi"("State In"=Process_State."Abort", "Mngr Action"=Process_Mngr."Run Step", "FP"=w281, "error in (no error)"=w279) -> ("error out"=w278:errorcluster)  [unwired: 10 in, 1 out]
              }
            }
          }
          frame True {
            n213 = Enqueue Element(queue=w286, element="Check Cartridge") -> (error out=w284:errorcluster)  [unwired: 2 in, 2 out]
            n214 = property on="Cart Test Array" class="Arr (strict)"("Value"=T12[] []) -> ()  [unwired: 2 in, 2 out]
          }
        }
      }
      event Value Change {
        n215 = event-data() -> ("NewVal"=w290:bool)  [unwired: 1 in]
        n216 = case shown="True" w290 {
          tunnel: w288 -> [_ _]
          tunnel: [w292 w300] -> w289
          tunnel: w288 -> [w291 _]
          tunnel: w287 -> [_ w302]
          frame False {
            n217 = flat-sequence {
              tunnel: w291 -> [w298]
              tunnel: [w295] -> w292
              frame #0 {
                n218 = global write "Main Globals.vi" "Cancel"(TRUE ("Cancel")) -> ()
              }
              frame #1 {
                n219 = global read "Hardware Globals.vi" "Zaber VISA"() -> (w297:refnum<visa-resource-name>)
                n220 = call "Stop.vi"("VISA resource name"=w297) -> ("error out"=w296:errorcluster)  [unwired: 9 in, 1 out]
                n221 = call "Process Mngr.vi"("State In"=Process_State."Abort", "Mngr Action"=Process_Mngr."Run Step", "FP"=w298, "error in (no error)"=w296) -> ("error out"=w295:errorcluster)  [unwired: 10 in, 1 out]
              }
            }
          }
          frame True {
            n222 = Enqueue Element(queue=w302, element="Rinse All Wells") -> (error out=w300:errorcluster)  [unwired: 2 in, 2 out]
          }
        }
      }
      event Value Change {
        n223 = event-data() -> ("NewVal"=w306:bool)  [unwired: 1 in]
        n224 = case shown="True" w306 {
          tunnel: w304 -> [_ _]
          tunnel: [w308 w316] -> w305
          tunnel: w304 -> [w307 _]
          tunnel: w303 -> [_ w318]
          frame False {
            n225 = flat-sequence {
              tunnel: w307 -> [w314]
              tunnel: [w311] -> w308
              frame #0 {
                n226 = global write "Main Globals.vi" "Cancel"(TRUE ("Cancel")) -> ()
              }
              frame #1 {
                n227 = global read "Hardware Globals.vi" "Zaber VISA"() -> (w313:refnum<visa-resource-name>)
                n228 = call "Stop.vi"("VISA resource name"=w313) -> ("error out"=w312:errorcluster)  [unwired: 9 in, 1 out]
                n229 = call "Process Mngr.vi"("State In"=Process_State."Abort", "Mngr Action"=Process_Mngr."Run Step", "FP"=w314, "error in (no error)"=w312) -> ("error out"=w311:errorcluster)  [unwired: 10 in, 1 out]
              }
            }
          }
          frame True {
            n230 = Enqueue Element(queue=w318, element="Fill Well") -> (error out=w316:errorcluster)  [unwired: 2 in, 2 out]
          }
        }
      }
      event Value Change {
        n231 = event-data() -> ("NewVal"=w322:bool)  [unwired: 1 in]
        n232 = case shown="True" w322 {
          tunnel: w320 -> [_ _]
          tunnel: [w324 w332] -> w321
          tunnel: w320 -> [w323 _]
          tunnel: w319 -> [_ w334]
          frame False {
            n233 = flat-sequence {
              tunnel: w323 -> [w330]
              tunnel: [w327] -> w324
              frame #0 {
                n234 = global write "Main Globals.vi" "Cancel"(TRUE ("Cancel")) -> ()
              }
              frame #1 {
                n235 = global read "Hardware Globals.vi" "Zaber VISA"() -> (w329:refnum<visa-resource-name>)
                n236 = call "Stop.vi"("VISA resource name"=w329) -> ("error out"=w328:errorcluster)  [unwired: 9 in, 1 out]
                n237 = call "Process Mngr.vi"("State In"=Process_State."Abort", "Mngr Action"=Process_Mngr."Run Step", "FP"=w330, "error in (no error)"=w328) -> ("error out"=w327:errorcluster)  [unwired: 10 in, 1 out]
              }
            }
          }
          frame True {
            n238 = Enqueue Element(queue=w334, element="Drain All Wells") -> (error out=w332:errorcluster)  [unwired: 2 in, 2 out]
          }
        }
      }
      event "Man Script Run": Value Change {
        n239 = event-data() -> ("NewVal"=w337:bool)  [unwired: 1 in]
        n240 = flat-sequence {
          tunnel: w337 -> [w340]
          tunnel: w338 -> [w341]
          tunnel: [w341] -> w336
          tunnel: [w340] -> w335
          tunnel: w336 -> [w343]
          tunnel: w335 -> [w342]
          frame #0 {
            n241 = global write "Main Globals.vi" "Cancel"(FALSE ("Cancel")) -> ()
          }
          frame #1 {
            n242 = case shown="True" w342 {
              tunnel: w343 -> [_ w345]
              frame False {
                n243 = global write "Main Globals.vi" "Cancel"(TRUE ("Cancel")) -> ()
              }
              frame True {
                n244 = Enqueue Element(queue=w345, element="Manual Script Start") -> ()  [unwired: 2 in, 3 out]
              }
            }
          }
        }
      }
      event "Pump Load Script": Value Change {
        n245 = event-data() -> ()  [unwired: 1 in, 1 out]
        n246 = Enqueue Element(queue=w347, element="Pump Load Script") -> ()  [unwired: 2 in, 3 out]
      }
      event "Pump Clear Script": Value Change {
        n247 = event-data() -> ()  [unwired: 1 in, 1 out]
        n248 = flat-sequence {
          frame #0 {
            n249 = local write "Pump Script Array"(T25[] [] ("Pump Script Array")) -> ()
          }
          frame #1 {
            n250 = local write "Pump Clear Script"(FALSE ("Pump Clear Script")) -> ()
          }
        }
      }
      event Value Change {
        n251 = event-data() -> ()  [unwired: 1 in, 1 out]
        n252 = Enqueue Element(queue=w351, element="Unlock Cart1") -> ()  [unwired: 2 in, 3 out]
      }
      event Value Change {
        n253 = event-data() -> ()  [unwired: 1 in, 1 out]
        n254 = Enqueue Element(queue=w353, element="Unlock Cart2") -> ()  [unwired: 2 in, 3 out]
      }
      event Value Change {
        n255 = event-data() -> ()  [unwired: 1 in, 1 out]
        n256 = Enqueue Element(queue=w355, element="Unlock Cart3") -> ()  [unwired: 2 in, 3 out]
      }
      event Value Change {
        n257 = event-data() -> ()  [unwired: 1 in, 1 out]
        n258 = Enqueue Element(queue=w357, element="Unlock Cart4") -> ()  [unwired: 2 in, 3 out]
      }
      event "Save Config": Value Change {
        n259 = event-data() -> ()  [unwired: 1 in, 1 out]
        n260 = Enqueue Element(queue=w363, element="Save Cfg") -> (error out=w361:errorcluster)  [unwired: 2 in, 2 out]
        n261 = local read "Config"() -> (w359:T1)
        n262 = call "Tecan Mngr.vi"("Mngr Action"=Tricon_Mngr."Set Config", "Pump Config"=w359, "error in (no error)"=w361) -> ()  [unwired: 7 in, 6 out]
      }
      event "Protocol Save": Value Change {
        n263 = event-data() -> ()  [unwired: 1 in, 1 out]
        n264 = Enqueue Element(queue=w365, element="Save Protocol") -> ()  [unwired: 2 in, 3 out]
      }
      event "Protocol Load": Value Change {
        n265 = event-data() -> ()  [unwired: 1 in, 1 out]
        n266 = Enqueue Element(queue=w367, element="Load Protocol") -> ()  [unwired: 2 in, 3 out]
      }
      event Value Change {
        n267 = event-data() -> ()  [unwired: 1 in, 1 out]
        n268 = Enqueue Element(queue=w369, element="Pump Init") -> ()  [unwired: 2 in, 3 out]
      }
      event "Manual Script Array": Value Change {
        n269 = event-data() -> ()  [unwired: 1 in, 1 out]
        n270 = local read "Manual Script Array"() -> (w372:T23[])
        n271 = Empty Array?(array=w372) -> (empty?=w371:bool)
        n272 = case shown="False" w371 {
          tunnel: w372 -> [w374 w379]
          tunnel: [w373 w379] -> w370
          frame False {
            n273 = for {
              tunnel: w374 -> [w378] mode=indexing
              tunnel: [w375] -> w373 mode=indexing
              i -> [w377]
              n274 = Increment(x=w377) -> (x+1=w376:i32)
              n275 = Bundle By Name(cluster=w378, "Step"=w376) -> (w375:T23)
            }
          }
          frame True {
          }
        }
        n276 = local write "Manual Script Array"(w370) -> ()
      }
    }
    n277 = call "Error Logger.vi"("Action"=T27."Update", "error in"=w57) -> ("error out"=w56:errorcluster)  [unwired: 8 in, 1 out]
  }
  "error out" <- w31
  n278 = while "State Machines" {
    tunnel: w21 -> [w388]
    tunnel: w14 -> [w384]
    tunnel: [w381] -> w30
    stop <- w387 stop-if-true
    n279 = Dequeue Element(queue=w388) -> (queue out=w380:refnum<queue>, element=w385:string, error out=w386:errorcluster)  [unwired: 2 in, 1 out]
    n280 = case shown="\"Init Process SM\"" w385 {
      selector: w385 -> [_ _ _ _ _ _ _ _ _ _ _ _ _ _ _ _ _ _ _ _ _ w570]
      tunnel: [_ _ _ _ _ _ _ _ _ _ _ _ _ _ _ _ _ _ _ _ TRUE TRUE] -> w387
      tunnel: w386 -> [w392 w405 w413 w416 w426 w434 w442 w450 w463 w473 w483 w494 w505 w515 w523 w532 w540 w548 w557 w565 w568 w573]
      tunnel: [w396 w401 w410 w415 w423 w432 w440 w448 w455 w467 w477 w488 w499 w509 w520 w528 w536 w545 w553 w561 w568 w573] -> w383
      tunnel: w384 -> [w390 w404 w407 w419 w425 w433 w441 w449 w462 w472 w482 w493 w504 w514 w518 w526 w535 w543 w551 w560 _ _]
      tunnel: w380 -> [w394 w400 w408 w420 _ _ _ _ _ _ _ _ _ _ _ _ _ _ _ _ _ _]
      frame "Init Process SM" {
        n281 = call "Process Mngr.vi"("Mngr Action"=Process_Mngr."Init", "FP"=w390, "error in (no error)"=w392) -> ("error out"=w391:errorcluster)  [unwired: 11 in, 1 out]
        n282 = Enqueue Element(queue=w394, element="Process SM", error in (no error)=w391) -> (error out=w396:errorcluster)  [unwired: 1 in, 2 out]
        n283 = Wait Until Next ms Multiple(millisecond multiple=u32 100) -> ()  [unwired: 1 out]
      }
      frame "Process SM" {
        n284 = call "Process Mngr.vi"("Mngr Action"=Process_Mngr."Update", "FP"=w404, "error in (no error)"=w405) -> ("error out"=w399:errorcluster)  [unwired: 11 in, 1 out]
        n285 = call "Error Logger.vi"("Action"=T27."Update", "error in"=w399) -> ("error out"=w398:errorcluster)  [unwired: 8 in, 1 out]
        n286 = Enqueue Element(queue=w400, element="Process SM", error in (no error)=w398) -> (error out=w401:errorcluster)  [unwired: 1 in, 2 out]
      }
      frame "Init Cartridge SM" {
        n287 = call "Cartridge Mngr.vi"("Main References"=w407, "Mngr Action"=Cartridge_Mngr."Init", "error in (no error)"=w413) -> ("error out"=w411:errorcluster)  [unwired: 6 in, 2 out]
        n288 = Enqueue Element(queue=w408, element="Cartridge SM", error in (no error)=w411) -> (error out=w410:errorcluster)  [unwired: 1 in, 2 out]
        n289 = Wait Until Next ms Multiple(millisecond multiple=u32 100) -> ()  [unwired: 1 out]
      }
      frame "Cartridge SM" {
        n290 = call "Cartridge Mngr.vi"("Main References"=w419, "Mngr Action"=Cartridge_Mngr."Update", "error in (no error)"=w416) -> ("error out"=w414:errorcluster)  [unwired: 6 in, 2 out]
        n291 = Enqueue Element(queue=w420, element="Cartridge SM", error in (no error)=w416) -> (error out=w421:errorcluster)  [unwired: 1 in, 2 out]
        n292 = Merge Errors(w421, w414) -> (w415:errorcluster)
        n293 = Wait Until Next ms Multiple(millisecond multiple=u32 100) -> ()  [unwired: 1 out]
      }
      frame "Unlock Cart1" {
        n294 = call "Cartridge Mngr.vi"("Main References"=w425, "Mngr Action"=Cartridge_Mngr."Unlock", "error in (no error)"=w426, "Cartrdige #"=1) -> ("error out"=w424:errorcluster)  [unwired: 5 in, 2 out]
        n295 = flat-sequence {
          tunnel: w424 -> [w430]
          tunnel: [w430] -> w423
          frame #0 {
            n296 = property on="Eject" class="Bool (strict)"("Value"=FALSE) -> ()  [unwired: 2 in, 2 out]
          }
        }
      }
      frame "Unlock Cart2" {
        n297 = call "Cartridge Mngr.vi"("Main References"=w433, "Mngr Action"=Cartridge_Mngr."Unlock", "error in (no error)"=w434, "Cartrdige #"=2) -> ("error out"=w431:errorcluster)  [unwired: 5 in, 2 out]
        n298 = flat-sequence {
          tunnel: [w438] -> w432
          tunnel: w431 -> [w438]
          frame #0 {
            n299 = property on="Eject" class="Bool (strict)"("Value"=FALSE) -> ()  [unwired: 2 in, 2 out]
          }
        }
      }
      frame "Unlock Cart3" {
        n300 = call "Cartridge Mngr.vi"("Main References"=w441, "Mngr Action"=Cartridge_Mngr."Unlock", "error in (no error)"=w442, "Cartrdige #"=3) -> ("error out"=w439:errorcluster)  [unwired: 5 in, 2 out]
        n301 = flat-sequence {
          tunnel: [w446] -> w440
          tunnel: w439 -> [w446]
          frame #0 {
            n302 = property on="Eject" class="Bool (strict)"("Value"=FALSE) -> ()  [unwired: 2 in, 2 out]
          }
        }
      }
      frame "Unlock Cart4" {
        n303 = call "Cartridge Mngr.vi"("Main References"=w449, "Mngr Action"=Cartridge_Mngr."Unlock", "error in (no error)"=w450, "Cartrdige #"=4) -> ("error out"=w447:errorcluster)  [unwired: 5 in, 2 out]
        n304 = flat-sequence {
          tunnel: [w454] -> w448
          tunnel: w447 -> [w454]
          frame #0 {
            n305 = property on="Eject" class="Bool (strict)"("Value"=FALSE) -> ()  [unwired: 2 in, 2 out]
          }
        }
      }
      frame "Run Process Step" {
        n306 = local read "Commands"() -> (w458:T8)
        n307 = Unbundle By Name(w458) -> ("State"=w457:T11)
        n308 = call "Process Mngr.vi"("State In"=w457, "Mngr Action"=Process_Mngr."Run Step", "FP"=w462, "error in (no error)"=w463) -> ("error out"=w460:errorcluster)  [unwired: 10 in, 1 out]
        n309 = call "Error Logger.vi"("Action"=T27."Update", "error in"=w460) -> ("error out"=w456:errorcluster)  [unwired: 8 in, 1 out]
        n310 = flat-sequence {
          tunnel: w456 -> [w465]
          tunnel: [w465] -> w455
          frame #0 {
            n311 = property on="Run State" class="Bool (strict)"("Value"=FALSE) -> ()  [unwired: 2 in, 2 out]
          }
        }
      }
      frame "Clean&Dry Cartridge" {
        n312 = call "Process Mngr.vi"("State In"=Process_State."-clean cartridge", "Mngr Action"=Process_Mngr."Run Step", "FP"=w472, "error in (no error)"=w473) -> ("error out"=w470:errorcluster)  [unwired: 10 in, 1 out]
        n313 = call "Error Logger.vi"("Action"=T27."Update", "error in"=w470) -> ("error out"=w468:errorcluster)  [unwired: 8 in, 1 out]
        n314 = flat-sequence {
          tunnel: w468 -> [w475]
          tunnel: [w475] -> w467
          frame #0 {
            w474 = FALSE ("Value")
            n315 = local write "Main Clean Cart"(w474) -> ()
            n316 = property on="Check for leaks" class="Bool (strict)"("Value"=w474) -> ()  [unwired: 2 in, 2 out]
          }
        }
      }
      frame "Check Cartridge" {
        n317 = call "Process Mngr.vi"("State In"=Process_State."-check cartridge", "Mngr Action"=Process_Mngr."Run Step", "FP"=w482, "error in (no error)"=w483) -> ("error out"=w480:errorcluster)  [unwired: 10 in, 1 out]
        n318 = call "Error Logger.vi"("Action"=T27."Update", "error in"=w480) -> ("error out"=w478:errorcluster)  [unwired: 8 in, 1 out]
        n319 = flat-sequence {
          tunnel: w478 -> [w485]
          tunnel: [w485] -> w477
          frame #0 {
            n320 = property on="Check for leaks" class="Bool (strict)"("Value"=FALSE) -> ()  [unwired: 2 in, 2 out]
          }
        }
      }
      frame "Rinse All Wells" {
        n321 = property on="Number of rinses" class="DigNum (strict)"() -> ("Value"=w486:dbl)  [unwired: 2 in, 2 out]
        n322 = call "Process Mngr.vi"("State In"=Process_State."-rinse wells", "Mngr Action"=Process_Mngr."Run Step", "FP"=w493, "Manual Input"=w486, "error in (no error)"=w494) -> ("error out"=w491:errorcluster)  [unwired: 9 in, 1 out]
        n323 = call "Error Logger.vi"("Action"=T27."Update", "error in"=w491) -> ("error out"=w489:errorcluster)  [unwired: 8 in, 1 out]
        n324 = flat-sequence {
          tunnel: w489 -> [w496]
          tunnel: [w496] -> w488
          frame #0 {
            n325 = property on="Rinse All Wells" class="Bool (strict)"("Value"=FALSE) -> ()  [unwired: 2 in, 2 out]
          }
        }
      }
      frame "Fill Well" {
        n326 = property on="Number of rinses" class="DigNum (strict)"() -> ("Value"=w497:dbl)  [unwired: 2 in, 2 out]
        n327 = call "Process Mngr.vi"("State In"=Process_State."-fill well", "Mngr Action"=Process_Mngr."Run Step", "FP"=w504, "Manual Input"=w497, "error in (no error)"=w505) -> ("error out"=w502:errorcluster)  [unwired: 9 in, 1 out]
        n328 = call "Error Logger.vi"("Action"=T27."Update", "error in"=w502) -> ("error out"=w500:errorcluster)  [unwired: 8 in, 1 out]
        n329 = flat-sequence {
          tunnel: w500 -> [w507]
          tunnel: [w507] -> w499
          frame #0 {
            n330 = property on="Fill" class="Bool (strict)"("Value"=FALSE) -> ()  [unwired: 2 in, 2 out]
          }
        }
      }
      frame "Drain All Wells" {
        n331 = call "Process Mngr.vi"("State In"=Process_State."-drain all", "Mngr Action"=Process_Mngr."Run Step", "FP"=w514, "error in (no error)"=w515) -> ("error out"=w512:errorcluster)  [unwired: 10 in, 1 out]
        n332 = call "Error Logger.vi"("Action"=T27."Update", "error in"=w512) -> ("error out"=w510:errorcluster)  [unwired: 8 in, 1 out]
        n333 = flat-sequence {
          tunnel: w510 -> [w517]
          tunnel: [w517] -> w509
          frame #0 {
            n334 = property on="Fill" class="Bool (strict)"("Value"=FALSE) -> ()  [unwired: 2 in, 2 out]
          }
        }
      }
      frame "Manual Script Start" {
        n335 = call "Scripting Mngr.vi"("Mngr Action"=Script_Mngr_Action."Run Script", "Main References"=w518, "error in (no error)"=w523, "Script Choice"=Script_Mngr_Script_choice."Manual Script") -> ("error out"=w521:errorcluster)  [unwired: 10 in, 1 out]
        n336 = flat-sequence {
          tunnel: w521 -> [w525]
          tunnel: [w525] -> w520
          frame #0 {
            w524 = FALSE ("Pump Load Script")
            n337 = local write "Man Script Run"(w524) -> ()
            n338 = global write "Main Globals.vi" "Stop Script"(w524) -> ()
            n339 = global write "Main Globals.vi" "Cancel"(w524) -> ()
          }
        }
      }
      frame "Manual Script Load" {
        n340 = call "Scripting Mngr.vi"("Mngr Action"=Script_Mngr_Action."Load Script", "Main References"=w526, "error in (no error)"=w532, "Script Choice"=Script_Mngr_Script_choice."Manual Script") -> ("selected path"=w527:path, "error out"=w529:errorcluster)  [unwired: 10 in]
        n341 = local write "Man Script Path"(w527) -> ()
        n342 = flat-sequence {
          tunnel: w529 -> [w534]
          tunnel: [w534] -> w528
          frame #0 {
            n343 = local write "Man Script Load"(FALSE ("Pump Load Script")) -> ()
          }
        }
      }
      frame "Manual Script Save" {
        n344 = call "Scripting Mngr.vi"("Mngr Action"=Script_Mngr_Action."Save Script", "Main References"=w535, "error in (no error)"=w540, "Script Choice"=Script_Mngr_Script_choice."Manual Script") -> ("error out"=w537:errorcluster)  [unwired: 10 in, 1 out]
        n345 = flat-sequence {
          tunnel: w537 -> [w542]
          tunnel: [w542] -> w536
          frame #0 {
            n346 = local write "Man Script Save"(FALSE ("Pump Save Script")) -> ()
          }
        }
      }
      frame "Pump Start Script" {
        n347 = call "Scripting Mngr.vi"("Mngr Action"=Script_Mngr_Action."Run Script", "Main References"=w543, "error in (no error)"=w548, "Script Choice"=Script_Mngr_Script_choice."Pump Script") -> ("error out"=w546:errorcluster)  [unwired: 10 in, 1 out]
        n348 = flat-sequence {
          tunnel: w546 -> [w550]
          tunnel: [w550] -> w545
          frame #0 {
            w549 = FALSE ("Pump Load Script")
            n349 = local write "Pump Start Script"(w549) -> ()
            n350 = global write "Main Globals.vi" "Stop Script"(w549) -> ()
            n351 = global write "Main Globals.vi" "Cancel"(w549) -> ()
          }
        }
      }
      frame "Pump Load Script" {
        n352 = call "Scripting Mngr.vi"("Mngr Action"=Script_Mngr_Action."Load Script", "Main References"=w551, "error in (no error)"=w557, "Script Choice"=Script_Mngr_Script_choice."Pump Script") -> ("selected path"=w552:path, "error out"=w554:errorcluster)  [unwired: 10 in]
        n353 = local write "Pump Script File"(w552) -> ()
        n354 = flat-sequence {
          tunnel: w554 -> [w559]
          tunnel: [w559] -> w553
          frame #0 {
            n355 = local write "Pump Load Script"(FALSE ("Pump Load Script")) -> ()
          }
        }
      }
      frame "Pump Save Script" {
        n356 = call "Scripting Mngr.vi"("Mngr Action"=Script_Mngr_Action."Save Script", "Main References"=w560, "error in (no error)"=w565, "Script Choice"=Script_Mngr_Script_choice."Pump Script") -> ("error out"=w562:errorcluster)  [unwired: 10 in, 1 out]
        n357 = flat-sequence {
          tunnel: w562 -> [w567]
          tunnel: [w567] -> w561
          frame #0 {
            n358 = local write "Pump Save Script"(FALSE ("Pump Save Script")) -> ()
          }
        }
      }
      frame "Quit" {
      }
      frame Default {
        n359 = Concatenate Strings("unkown queue msg:\n" ("string"), w570) -> (w571:string)
        n360 = One Button Dialog(message=w571) -> ()  [unwired: 1 in, 1 out]
      }
    }
    n361 = call "Error Logger.vi"("Action"=T27."Update", "error in"=w383) -> ("error out"=w381:errorcluster)  [unwired: 8 in, 1 out]
  }
  n362 = while "Events Handler" {
    tunnel: w26 -> [w585]
    tunnel: w14 -> [w582]
    tunnel: [w578] -> w35
    tunnel: w21 -> [w576]
    tunnel: w8 -> [w575]
    stop <- w581 stop-if-true
    n363 = Dequeue Element(queue=w585) -> (queue out=w580:refnum<queue>, element=w584:string, error out=w583:errorcluster)  [unwired: 2 in, 1 out]
    n364 = case shown="Default" w584 {
      selector: w584 -> [_ _ _ _ _ _ _ _ _ _ _ _ _ _ _ _ _ _ _ _ _ _ _ _ _ _ _ _ _ _ _ _ _ _ w1071 _]
      tunnel: w583 -> [w590 w631 w635 w666 w674 w683 w692 w705 w770 w778 w788 w810 w814 w833 w838 w848 w860 w874 w891 w908 w925 w942 w952 w965 w974 w983 w992 w1000 w1015 w1029 w1044 w1053 w1059 w1066 w1070 w1076]
      tunnel: [w590 w618 w634 w658 w667 w680 w688 w695 w766 w773 w782 w800 w817 w831 w836 w841 w857 w867 w885 w902 w920 w935 w950 w964 w973 w982 w991 w1009 w1014 w1026 w1037 w1051 w1057 w1061 w1070 w1086] -> w579
      tunnel: w582 -> [_ _ _ w657 w673 w682 w691 _ _ _ _ _ _ _ _ _ _ _ _ _ _ _ _ _ _ _ _ _ _ _ _ _ _ _ _ _]
      tunnel: [_ _ _ _ _ _ _ _ FALSE FALSE FALSE FALSE FALSE _ FALSE _ _ _ _ _ _ _ _ FALSE FALSE FALSE FALSE FALSE FALSE FALSE FALSE FALSE FALSE FALSE _ TRUE] -> w581
      tunnel: w580 -> [_ _ w632 _ _ _ _ w706 w765 _ _ _ _ _ _ _ _ _ _ _ _ _ _ _ _ _ _ _ _ _ _ _ _ _ _ _]
      tunnel: w576 -> [_ _ _ _ _ _ _ _ _ _ _ _ _ w830 _ _ _ _ _ _ _ _ _ _ _ _ _ _ _ _ _ _ _ _ _ _]
      tunnel: w575 -> [_ _ _ _ _ _ _ _ _ _ w784 _ _ _ _ _ _ _ _ _ _ _ _ _ _ _ _ _ _ _ _ _ _ _ _ _]
      frame "Init" {
        n365 = Current VI's Path() -> (path=w591:path)
        "Root path" <- w591
        n366 = call <userlib>:"MGI Is Runtime.vi"() -> ("Run Time System?"=w611:bool)  [unwired: 7 in]
        "Run Time System?" <- w611
        n367 = case shown="True" w611 {
          tunnel: w591 -> [w614 w617]
          tunnel: [w612 w615] -> w587
          frame True {
            n368 = Strip Path(path=w614) -> (stripped path=w613:path)  [unwired: 1 out]
            n369 = Strip Path(path=w613) -> (stripped path=w612:path)  [unwired: 1 out]
          }
          frame False {
            n370 = Strip Path(path=w617) -> (stripped path=w616:path)  [unwired: 1 out]
            n371 = Strip Path(path=w616) -> (stripped path=w615:path)  [unwired: 1 out]
          }
        }
        n372 = Build Path(base path=w587, name or relative path="Python") -> (appended path=w595:path)
        n373 = Build Path(base path=w587, name or relative path="Data") -> (appended path=w603:path)
        n374 = Build Path(base path=w587, name or relative path="Logs") -> (appended path=w604:path)
        n375 = Build Path(base path=w587, name or relative path="Scripts") -> (appended path=w605:path)
        n376 = Build Path(base path=w587, name or relative path="Config") -> (appended path=w606:path)
        n377 = Build Path(base path=w587, name or relative path="Protocols") -> (appended path=w597:path)
        n378 = Build Path(base path=w587, name or relative path="Reports") -> (appended path=w588:path)
        n379 = property on="Syringe Pump" class="Clust (strict)"("DisabledEnum"=T26."Disabled and Grayed Out" ("Disabled")) -> ()  [unwired: 2 in, 2 out]
        n380 = call "Create Folder If Misssing.vi"("Path In"=w595) -> ("Path Out"=w593:path)  [unwired: 1 in, 1 out]
        "Python Folder" <- w593
        n381 = call "Create Folder If Misssing.vi"("Path In"=w603) -> ("Path Out"=w592:path)  [unwired: 1 in, 1 out]
        "Data Folder" <- w592
        n382 = call "Create Folder If Misssing.vi"("Path In"=w604) -> ("Path Out"=w601:path)  [unwired: 1 in, 1 out]
        "Logs Folder" <- w601
        n383 = call "Create Folder If Misssing.vi"("Path In"=w605) -> ("Path Out"=w602:path)  [unwired: 1 in, 1 out]
        "Scripts Folder" <- w602
        n384 = call "Create Folder If Misssing.vi"("Path In"=w606) -> ("Path Out"=w600:path)  [unwired: 1 in, 1 out]
        "Config Folder" <- w600
        n385 = call "Create Folder If Misssing.vi"("Path In"=w597) -> ("Path Out"=w598:path)  [unwired: 1 in, 1 out]
        "Protocols Folder" <- w598
        n386 = call "Create Folder If Misssing.vi"("Path In"=w588) -> ("Path Out"=w586:path)  [unwired: 1 in, 1 out]
        "Reports" <- w586
        n387 = global write "Main Globals.vi" "Python Folder"(w593) -> ()
        n388 = global write "Main Globals.vi" "Data Folder"(w592) -> ()
        n389 = global write "Main Globals.vi" "Logs Folder"(w601) -> ()
        n390 = global write "Main Globals.vi" "Scripts Folder"(w602) -> ()
        n391 = global write "Main Globals.vi" "Config Folder"(w600) -> ()
        n392 = global write "Main Globals.vi" "Protocol Folder"(w598) -> ()
        n393 = global write "Main Globals.vi" "Reports"(w586) -> ()
      }
      frame "Init Loggers" {
        n394 = global read "Main Globals.vi" "Logs Folder"() -> (w622:path)
        n395 = Build Path(base path=w622, name or relative path="Error Log.dat") -> (appended path=w625:path)
        n396 = call "Error Logger.vi"("Action"=T27."Init", "error in"=w631, "Log File"=w625) -> ("error out"=w630:errorcluster)  [unwired: 7 in, 1 out]
        n397 = Build Path(base path=w622, name or relative path="Main Status Log.dat") -> (appended path=w624:path)
        n398 = call "Main Status Logger.vi"("Action"=T27."Init", "error in"=w630, "Log File"=w624) -> ("error out"=w623:errorcluster)  [unwired: 7 in, 1 out]
        n399 = Build Path(base path=w622, name or relative path="Error Log.dat") -> (appended path=w620:path)
        n400 = call "Error Logger.vi"("Action"=T27."Init", "error in"=w623, "Log File"=w620) -> ("error out"=w618:errorcluster)  [unwired: 7 in, 1 out]
      }
      frame "Init FrontPanel" {
        n401 = local read "Zaber Found"() -> (w640:bool)
        n402 = local read "Relays Found"() -> (w639:bool)
        n403 = local read "NI DAQ Found"() -> (w638:bool)
        n404 = local read "Pump Found"() -> (w637:bool)
        n405 = local read "Valco Found"() -> (w636:bool)
        n406 = Compound Arithmetic op=AND(w640, w639, w638, w637, w636) -> (w633:bool)
        n407 = case shown="True" w633 {
          tunnel: w635 -> [w642 w651]
          tunnel: [w642 w650] -> w634
          tunnel: w632 -> [_ w649]
          frame False {
            n408 = local read "Cartridges"() -> (w644:T6)
            n409 = Bundle By Name(cluster=w644, "Current Status"="System has failed to initialize") -> (w641:T6)
            n410 = local write "Cartridges"(w641) -> ()
          }
          frame True {
            n411 = local read "Cartridges"() -> (w647:T6)
            n412 = Bundle By Name(cluster=w647, "Current Status"="System is  initialized") -> (w646:T6)
            n413 = Enqueue Element(queue=w649, element="Start SMs", error in (no error)=w651) -> (error out=w650:errorcluster)  [unwired: 1 in, 2 out]
            n414 = local write "Cartridges"(w646) -> ()
          }
        }
      }
      frame "Load Cfg" {
        n415 = global read "Main Globals.vi" "Config Folder"() -> (w664:path)
        n416 = Build Path(base path=w664, name or relative path="Config.ini") -> (appended path=w660:path)
        n417 = call "Config Mngr.vi"("Main References"=w657, "Mngr Action"=Config_Mngr."Load Config", "error in"=w666, "path"=w660) -> ("error out"=w656:errorcluster, "Config"=w661:T1)  [unwired: 5 in, 1 out]
        n418 = Unbundle By Name(w661) -> ("Full Stroke (cnts)"=w662:i32, "Default Protocol"=w653:path)
        n419 = global read "Main Globals.vi" "Protocol Folder"() -> (w655:path)
        n420 = Path To String(path=w653) -> (string=w652:string)
        n421 = Build Path(base path=w655, name or relative path=w653) -> (appended path=w654:path)
        n422 = global write "Hardware Globals.vi" "Pump Cnts"(w662) -> ()
        n423 = local write "Current Protocol"(w652) -> ()
        n424 = call "Config Mngr.vi"("Main References"=w657, "Mngr Action"=Config_Mngr."Load Protocol", "error in"=w656, "path"=w654) -> ("error out"=w658:errorcluster)  [unwired: 5 in, 2 out]
      }
      frame "Save Cfg" {
        n425 = global read "Main Globals.vi" "Config Folder"() -> (w670:path)
        n426 = Build Path(base path=w670, name or relative path="Config.ini") -> (appended path=w669:path)
        n427 = call "Config Mngr.vi"("Main References"=w673, "Mngr Action"=Config_Mngr."Save Config", "error in"=w674, "path"=w669) -> ("error out"=w668:errorcluster)  [unwired: 5 in, 2 out]
        n428 = flat-sequence {
          tunnel: w668 -> [w675]
          tunnel: [w675] -> w667
          frame #0 {
            n429 = local write "Save Config"(FALSE ("Save Config")) -> ()
          }
        }
      }
      frame "Save Protocol" {
        n430 = call "Config Mngr.vi"("Main References"=w682, "Mngr Action"=Config_Mngr."Save Protocol", "error in"=w683) -> ("error out"=w677:errorcluster, "path out"=w679:path)  [unwired: 6 in, 1 out]
        n431 = Strip Path(path=w679) -> (name=w678:string)  [unwired: 1 out]
        n432 = local write "Current Protocol"(w678) -> ()
        n433 = flat-sequence {
          tunnel: w677 -> [w684]
          tunnel: [w684] -> w680
          frame #0 {
            n434 = local write "Protocol Save"(FALSE ("Save Config")) -> ()
          }
        }
      }
      frame "Load Protocol" {
        n435 = call "Config Mngr.vi"("Main References"=w691, "Mngr Action"=Config_Mngr."Load Protocol", "error in"=w692) -> ("error out"=w689:errorcluster, "path out"=w686:path)  [unwired: 6 in, 1 out]
        n436 = Strip Path(path=w686) -> (name=w687:string)  [unwired: 1 out]
        n437 = local write "Current Protocol"(w687) -> ()
        n438 = flat-sequence {
          tunnel: w689 -> [w693]
          tunnel: [w693] -> w688
          frame #0 {
            n439 = local write "Protocol Load"(FALSE ("Save Config")) -> ()
          }
        }
      }
      frame "Init Hardware" {
        n440 = case shown="True" TRUE {
          tunnel: w705 -> [w732 w737]
          tunnel: w706 -> [w731 w735]
          tunnel: [w731 w734] -> w704
          tunnel: [w732 w733] -> w703
          frame False {
          }
          frame True {
            n441 = Enqueue Element(queue=w735, element="DAQ Connect", error in (no error)=w737) -> (queue out=w734:refnum<queue>, error out=w733:errorcluster)  [unwired: 1 in, 1 out]
          }
        }
        n442 = case shown="True" TRUE {
          tunnel: w703 -> [w753 w758]
          tunnel: w704 -> [w752 w756]
          tunnel: [w752 w755] -> w713
          tunnel: [w753 w754] -> w712
          frame False {
          }
          frame True {
            n443 = Enqueue Element(queue=w756, element="Relay Connect", error in (no error)=w758) -> (queue out=w755:refnum<queue>, error out=w754:errorcluster)  [unwired: 1 in, 1 out]
          }
        }
        n444 = case shown="True" TRUE {
          tunnel: w713 -> [w746 w750]
          tunnel: w712 -> [w745 w749]
          tunnel: [w746 w748] -> w711
          tunnel: [w745 w747] -> w710
          frame False {
          }
          frame True {
            n445 = Enqueue Element(queue=w750, element="Valco Connect", error in (no error)=w749) -> (queue out=w748:refnum<queue>, error out=w747:errorcluster)  [unwired: 1 in, 1 out]
          }
        }
        n446 = case shown="True" TRUE {
          tunnel: w711 -> [w738 w743]
          tunnel: w710 -> [w739 w742]
          tunnel: [w739 w741] -> w701
          tunnel: [w738 w740] -> w700
          frame False {
          }
          frame True {
            n447 = Enqueue Element(queue=w743, element="Pump Connect", error in (no error)=w742) -> (queue out=w740:refnum<queue>, error out=w741:errorcluster)  [unwired: 1 in, 1 out]
          }
        }
        n448 = case shown="True" TRUE {
          tunnel: w701 -> [w725 w730]
          tunnel: w700 -> [w724 w728]
          tunnel: [w724 w727] -> w697
          tunnel: [w725 w726] -> w696
          frame False {
          }
          frame True {
            n449 = Enqueue Element(queue=w728, element="Zaber Connect", error in (no error)=w730) -> (queue out=w727:refnum<queue>, error out=w726:errorcluster)  [unwired: 1 in, 1 out]
          }
        }
        n450 = case shown="False" FALSE {
          tunnel: w696 -> [w718 w723]
          tunnel: w697 -> [w716 w721]
          tunnel: [w715 w720] -> _
          tunnel: [w714 w719] -> w695
          frame True {
            n451 = Enqueue Element(queue=w716, element="Start SMs", error in (no error)=w718) -> (queue out=w715:refnum<queue>, error out=w714:errorcluster)  [unwired: 1 in, 1 out]
          }
          frame False {
            n452 = Enqueue Element(queue=w721, element="Init FrontPanel", error in (no error)=w723) -> (queue out=w720:refnum<queue>, error out=w719:errorcluster)  [unwired: 1 in, 1 out]
          }
        }
      }
      frame "Pump Connect" {
        n453 = local read "Config"() -> (w759:T1)
        n454 = call "Tecan Mngr.vi"("Address"=u8 1, "Mngr Action"=Tricon_Mngr."Init COM", "Pump Config"=w759, "error in (no error)"=w770) -> ("Connected"=w761:bool, "error out"=w767:errorcluster)  [unwired: 6 in, 4 out]
        n455 = Select(t=T26."Enabled" ("Disabled"), s=w761, f=T26."Disabled and Grayed Out" ("Disabled")) -> (s? t:f=w760:T26)
        n456 = local write "Pump Found"(w761) -> ()
        n457 = property on="Syringe Pump" class="Clust (strict)"("DisabledEnum"=w760) -> ()  [unwired: 2 in, 2 out]
        n458 = Enqueue Element(queue=w765, element="Pump Init", error in (no error)=w767) -> (error out=w766:errorcluster)  [unwired: 1 in, 2 out]
      }
      frame "Valco Connect" {
        n459 = call "Valco Valve Mngr.vi"("Mngr Action"=Valco_Valve_Mngr_Action."Connect", "error in (no error)"=w778) -> ("Connected"=w775:bool, "error out"=w773:errorcluster)  [unwired: 9 in, 3 out]
        n460 = Select(t=T26."Enabled" ("Disabled"), s=w775, f=T26."Disabled and Grayed Out" ("Disabled")) -> (s? t:f=w772:T26)
        n461 = local write "Valco Found"(w775) -> ()
        n462 = property on="Man Valco" class="RadioBtnsControl (strict)"("DisabledEnum"=w772) -> ()  [unwired: 2 in, 2 out]
      }
      frame "DAQ Connect" {
        n463 = call "Timer Count 1 with Error Handling.vi"("Reset"=TRUE, "error in (no error)"=w788) -> ("error out"=w787:errorcluster)  [unwired: 6 in, 3 out]
        n464 = call "DAQ Manager.vi"("DAQ Name"="USB-6001", "DAQ Mngr Action"=DAQ_Mngr."Init", "error in (no error)"=w787) -> ("Connected"=w783:bool, "error out"=w785:errorcluster)  [unwired: 6 in, 5 out]
        n465 = Select(t=T26."Enabled" ("Disabled"), s=w783, f=T26."Disabled and Grayed Out" ("Disabled")) -> (s? t:f=w790:T26)
        n466 = case shown="True" w783 {
          tunnel: w785 -> [w795 w799]
          tunnel: [w795 w798] -> w781
          tunnel: w784 -> [_ w797]
          frame False {
          }
          frame True {
            n467 = Enqueue Element(queue=w797, element="Read Pressure", error in (no error)=w799) -> (error out=w798:errorcluster)  [unwired: 1 in, 2 out]
          }
        }
        n468 = local write "NI DAQ Found"(w783) -> ()
        n469 = property on="Man Cart Control" class="Clust (strict)"("DisabledEnum"=w790) -> ()  [unwired: 2 in, 2 out]
        n470 = property on="Cart Sense Cluster" class="Clust (strict)"("DisabledEnum"=w790) -> ()  [unwired: 2 in, 2 out]
        n471 = call "DAQ Manager.vi"("DAQ Mngr Action"=DAQ_Mngr."Pinch Valve Disengage", "error in (no error)"=w781) -> ("error out"=w782:errorcluster)  [unwired: 7 in, 6 out]
      }
      frame "Zaber Connect" {
        n472 = call "Zaber Manager.vi"("Action"=Mot_Stage_Mngr."Connect", "error in (no error)"=w810) -> ("Connected"=w807:bool, "error out"=w804:errorcluster)  [unwired: 7 in, 5 out]
        n473 = Select(t=T26."Enabled" ("Disabled"), s=w807, f=T26."Disabled and Grayed Out" ("Disabled")) -> (s? t:f=w803:T26)
        n474 = local write "Zaber Found"(w807) -> ()
        n475 = call "Zaber Manager.vi"("Action"=Mot_Stage_Mngr."Init", "error in (no error)"=w804) -> ("error out"=w801:errorcluster)  [unwired: 7 in, 6 out]
        n476 = property on="Motor Cluster" class="Clust (strict)"("DisabledEnum"=w803) -> ()  [unwired: 2 in, 2 out]
        n477 = call "Zaber Manager.vi"("Action"=Mot_Stage_Mngr."Home", "error in (no error)"=w801) -> ("error out"=w800:errorcluster)  [unwired: 7 in, 6 out]
      }
      frame "Relay Connect" {
        n478 = call "Denkovi Manager.vi"("Action"=Denkovi_Mngr."Search", "error in (no error)"=w814) -> ("error out"=w813:errorcluster)  [unwired: 7 in, 2 out]
        n479 = call "Denkovi Manager.vi"("Action"=Denkovi_Mngr."Init", "error in (no error)"=w813) -> ("error out"=w821:errorcluster, "Connected"=w824:bool)  [unwired: 7 in, 1 out]
        n480 = Select(t=T26."Enabled" ("Disabled"), s=w824, f=T26."Disabled and Grayed Out" ("Disabled")) -> (s? t:f=w823:T26)
        n481 = local write "Relays Found"(w824) -> ()
        n482 = property on="Man Peristaltic Ctrl" class="Bool (strict)"("DisabledEnum"=w823) -> ()  [unwired: 2 in, 2 out]
        n483 = call "Denkovi Manager.vi"("Action"=Denkovi_Mngr."Set All Relays", "error in (no error)"=w821, "Relays In"=bool[] [FALSE, FALSE, FALSE, FALSE, FALSE, FALSE, FALSE, TRUE, FALSE, FALSE, FALSE, FALSE, FALSE, FALSE, FALSE, FALSE]) -> ("error out"=w818:errorcluster)  [unwired: 6 in, 2 out]
        n484 = call "Denkovi Manager.vi"("Action"=Denkovi_Mngr."Vent&Close", "error in (no error)"=w818, "Relays In"=bool[] [TRUE, TRUE, TRUE, TRUE]) -> ("error out"=w817:errorcluster)  [unwired: 6 in, 2 out]
      }
      frame "Start SMs" {
        n485 = Enqueue Element(queue=w830, element="Init Cartridge SM", error in (no error)=w833) -> (error out=w832:errorcluster)  [unwired: 1 in, 2 out]
        n486 = Enqueue Element(queue=w830, element="Init Process SM", error in (no error)=w832) -> (error out=w831:errorcluster)  [unwired: 1 in, 2 out]
      }
      frame "Valco Set" {
        n487 = local read "Man Valco"() -> (w835:enum32{"Port1", "Port2", "Port3", "Port4"})
        n488 = To Byte Integer(number=w835) -> (8bit integer=w834:i8)
        n489 = call "Valco Valve Mngr.vi"("Valve"=w834, "Mngr Action"=Valco_Valve_Mngr_Action."Set Valve", "error in (no error)"=w838) -> ("error out"=w836:errorcluster)  [unwired: 8 in, 4 out]
      }
      frame "Zaber Abs Move" {
        n490 = local read "Motor Cluster"() -> (w844:T21)
        n491 = Unbundle By Name(w844) -> ("Mot Abs Dist"=w847:dbl)
        n492 = call "Zaber Manager.vi"("Action"=Mot_Stage_Mngr."Abs Move", "Value"=w847, "error in (no error)"=w848) -> ("error out"=w845:errorcluster)  [unwired: 6 in, 6 out]
        n493 = call "Zaber Manager.vi"("Action"=Mot_Stage_Mngr."Current Pos", "error in (no error)"=w845) -> ("Position(um)"=w843:dbl, "Position(cnts)"=w840:i64, "error out"=w842:errorcluster)  [unwired: 7 in, 4 out]
        n494 = flat-sequence {
          tunnel: w844 -> [w855]
          tunnel: w843 -> [w854]
          tunnel: w842 -> [w852]
          tunnel: [w852] -> w841
          tunnel: w840 -> [w850]
          frame #0 {
            n495 = Bundle By Name(cluster=w855, "Position(cnts)"=w850, "Position(mm)"=w854, "Mot Abs Move"=FALSE) -> (w853:T21)
            n496 = local write "Motor Cluster"(w853) -> ()
          }
        }
      }
      frame "Zaber Set Vel" {
        n497 = local read "Motor Cluster"() -> (w858:T21)
        n498 = Unbundle By Name(w858) -> ("Mot Max Vel"=w859:dbl)
        n499 = call "Zaber Manager.vi"("Action"=Mot_Stage_Mngr."Set Max Vel", "Value"=w859, "error in (no error)"=w860) -> ("error out"=w856:errorcluster)  [unwired: 6 in, 6 out]
        n500 = flat-sequence {
          tunnel: w858 -> [w865]
          tunnel: w856 -> [w863]
          tunnel: [w863] -> w857
          frame #0 {
            n501 = Bundle By Name(cluster=w865, "Mot Change Vel"=FALSE ("Mot Abs Move")) -> (w864:T21)
            n502 = local write "Motor Cluster"(w864) -> ()
          }
        }
      }
      frame "Zaber Rel Move+" {
        n503 = local read "Motor Cluster"() -> (w870:T21)
        n504 = Unbundle By Name(w870) -> ("Mot Rel Dist"=w873:dbl)
        n505 = call "Zaber Manager.vi"("Action"=Mot_Stage_Mngr."Rel Move", "Value"=w873, "error in (no error)"=w874) -> ("error out"=w871:errorcluster)  [unwired: 6 in, 6 out]
        n506 = call "Zaber Manager.vi"("Action"=Mot_Stage_Mngr."Current Pos", "error in (no error)"=w871) -> ("Position(um)"=w869:dbl, "Position(cnts)"=w866:i64, "error out"=w868:errorcluster)  [unwired: 7 in, 4 out]
        n507 = flat-sequence {
          tunnel: w870 -> [w881]
          tunnel: w869 -> [w880]
          tunnel: w868 -> [w878]
          tunnel: [w878] -> w867
          tunnel: w866 -> [w876]
          frame #0 {
            n508 = Bundle By Name(cluster=w881, "Position(cnts)"=w876, "Position(mm)"=w880, "Mot Rel +"=FALSE ("Mot Abs Move")) -> (w879:T21)
            n509 = local write "Motor Cluster"(w879) -> ()
          }
        }
      }
      frame "Zaber TW_pos" {
        n510 = local read "Config"() -> (w884:T1)
        n511 = Unbundle By Name(w884) -> ("TW Position"=w890:dbl)
        n512 = call "Zaber Manager.vi"("Action"=Mot_Stage_Mngr."Abs Move", "Value"=w890, "error in (no error)"=w891) -> ("error out"=w888:errorcluster)  [unwired: 6 in, 6 out]
        n513 = local read "Motor Cluster"() -> (w883:T21)
        n514 = call "Zaber Manager.vi"("Action"=Mot_Stage_Mngr."Current Pos", "error in (no error)"=w888) -> ("Position(um)"=w887:dbl, "Position(cnts)"=w882:i64, "error out"=w886:errorcluster)  [unwired: 7 in, 4 out]
        n515 = flat-sequence {
          tunnel: w883 -> [w898]
          tunnel: w887 -> [w897]
          tunnel: w886 -> [w895]
          tunnel: [w895] -> w885
          tunnel: w882 -> [w893]
          frame #0 {
            n516 = Bundle By Name(cluster=w898, "Position(cnts)"=w893, "Position(mm)"=w897) -> (w896:T21)
            n517 = local write "Motor Cluster"(w896) -> ()
            n518 = local write "Zaber TW_pos"(FALSE ("Zaber TW_pos")) -> ()
          }
        }
      }
      frame "Zaber Load_pos" {
        n519 = local read "Config"() -> (w901:T1)
        n520 = Unbundle By Name(w901) -> ("Load Position"=w907:dbl)
        n521 = call "Zaber Manager.vi"("Action"=Mot_Stage_Mngr."Abs Move", "Value"=w907, "error in (no error)"=w908) -> ("error out"=w905:errorcluster)  [unwired: 6 in, 6 out]
        n522 = local read "Motor Cluster"() -> (w900:T21)
        n523 = call "Zaber Manager.vi"("Action"=Mot_Stage_Mngr."Current Pos", "error in (no error)"=w905) -> ("Position(um)"=w904:dbl, "Position(cnts)"=w899:i64, "error out"=w903:errorcluster)  [unwired: 7 in, 4 out]
        n524 = flat-sequence {
          tunnel: w900 -> [w915]
          tunnel: w904 -> [w911]
          tunnel: w903 -> [w913]
          tunnel: [w913] -> w902
          tunnel: w899 -> [w910]
          frame #0 {
            n525 = Bundle By Name(cluster=w915, "Position(mm)"=w911, "Position(cnts)"=w910) -> (w914:T21)
            n526 = local write "Motor Cluster"(w914) -> ()
            n527 = local write "Zaber Load_pos"(FALSE ("Zaber TW_pos")) -> ()
          }
        }
      }
      frame "Zaber Bottom_pos" {
        n528 = local read "Config"() -> (w919:T1)
        n529 = Unbundle By Name(w919) -> ("Bottom Position"=w924:dbl)
        n530 = call "Zaber Manager.vi"("Action"=Mot_Stage_Mngr."Abs Move", "Value"=w924, "error in (no error)"=w925) -> ("error out"=w922:errorcluster)  [unwired: 6 in, 6 out]
        n531 = local read "Motor Cluster"() -> (w918:T21)
        n532 = call "Zaber Manager.vi"("Action"=Mot_Stage_Mngr."Current Pos", "error in (no error)"=w922) -> ("Position(um)"=w917:dbl, "Position(cnts)"=w916:i64, "error out"=w921:errorcluster)  [unwired: 7 in, 4 out]
        n533 = flat-sequence {
          tunnel: w918 -> [w930]
          tunnel: w921 -> [w932]
          tunnel: [w932] -> w920
          tunnel: w917 -> [w929]
          tunnel: w916 -> [w928]
          frame #0 {
            n534 = Bundle By Name(cluster=w930, "Position(mm)"=w929, "Position(cnts)"=w928) -> (w927:T21)
            n535 = local write "Motor Cluster"(w927) -> ()
            n536 = local write "Zaber Bottom_pos"(FALSE ("Zaber TW_pos")) -> ()
          }
        }
      }
      frame "Zaber Rel Move-" {
        n537 = local read "Motor Cluster"() -> (w938:T21)
        n538 = Unbundle By Name(w938) -> ("Mot Rel Dist"=w941:dbl)
        n539 = Negate(x=w941) -> (-x=w934:dbl)
        n540 = call "Zaber Manager.vi"("Action"=Mot_Stage_Mngr."Rel Move", "Value"=w934, "error in (no error)"=w942) -> ("error out"=w939:errorcluster)  [unwired: 6 in, 6 out]
        n541 = call "Zaber Manager.vi"("Action"=Mot_Stage_Mngr."Current Pos", "error in (no error)"=w939) -> ("Position(um)"=w937:dbl, "Position(cnts)"=w933:i64, "error out"=w936:errorcluster)  [unwired: 7 in, 4 out]
        n542 = flat-sequence {
          tunnel: w938 -> [w949]
          tunnel: w937 -> [w948]
          tunnel: w936 -> [w946]
          tunnel: [w946] -> w935
          tunnel: w933 -> [w944]
          frame #0 {
            n543 = Bundle By Name(cluster=w949, "Position(cnts)"=w944, "Position(mm)"=w948, "Mot Rel -"=FALSE ("Mot Abs Move")) -> (w947:T21)
            n544 = local write "Motor Cluster"(w947) -> ()
          }
        }
      }
      frame "Zaber Home" {
        n545 = call "Zaber Manager.vi"("Action"=Mot_Stage_Mngr."Home", "error in (no error)"=w952) -> ("error out"=w951:errorcluster)  [unwired: 7 in, 6 out]
        n546 = flat-sequence {
          tunnel: w951 -> [w954]
          tunnel: [w954] -> w950
          frame #0 {
            n547 = local read "Motor Cluster"() -> (w955:T21)
            n548 = Bundle By Name(cluster=w955, "Mot Home"=FALSE) -> (w956:T21)
            n549 = local write "Motor Cluster"(w956) -> ()
          }
        }
      }
      frame "DAQ Toggle Cart1" {
        n550 = local read "Man Cart Control"() -> (w963:T16)
        n551 = Unbundle By Name(w963) -> ("Cart1"=w960:bool)
        n552 = Select(t=DAQ_Mngr."Lock Cartridge" ("DAQ Mngr Action"), s=w960, f=DAQ_Mngr."Unlock Cartridge" ("DAQ Mngr Action")) -> (s? t:f=w959:T38)
        n553 = call "DAQ Manager.vi"("DAQ Mngr Action"=w959, "Value"=1.0, "error in (no error)"=w965) -> ("error out"=w964:errorcluster)  [unwired: 6 in, 6 out]
      }
      frame "DAQ Toggle Cart2" {
        n554 = local read "Man Cart Control"() -> (w972:T16)
        n555 = Unbundle By Name(w972) -> ("Cart2"=w969:bool)
        n556 = Select(t=DAQ_Mngr."Lock Cartridge" ("DAQ Mngr Action"), s=w969, f=DAQ_Mngr."Unlock Cartridge" ("DAQ Mngr Action")) -> (s? t:f=w968:T38)
        n557 = call "DAQ Manager.vi"("DAQ Mngr Action"=w968, "Value"=2.0, "error in (no error)"=w974) -> ("error out"=w973:errorcluster)  [unwired: 6 in, 6 out]
      }
      frame "DAQ Toggle Cart3" {
        n558 = local read "Man Cart Control"() -> (w981:T16)
        n559 = Unbundle By Name(w981) -> ("Cart3"=w978:bool)
        n560 = Select(t=DAQ_Mngr."Lock Cartridge" ("DAQ Mngr Action"), s=w978, f=DAQ_Mngr."Unlock Cartridge" ("DAQ Mngr Action")) -> (s? t:f=w977:T38)
        n561 = call "DAQ Manager.vi"("DAQ Mngr Action"=w977, "Value"=3.0, "error in (no error)"=w983) -> ("error out"=w982:errorcluster)  [unwired: 6 in, 6 out]
      }
      frame "DAQ Toggle Cart4" {
        n562 = local read "Man Cart Control"() -> (w990:T16)
        n563 = Unbundle By Name(w990) -> ("Cart4"=w987:bool)
        n564 = Select(t=DAQ_Mngr."Lock Cartridge" ("DAQ Mngr Action"), s=w987, f=DAQ_Mngr."Unlock Cartridge" ("DAQ Mngr Action")) -> (s? t:f=w986:T38)
        n565 = call "DAQ Manager.vi"("DAQ Mngr Action"=w986, "Value"=4.0, "error in (no error)"=w992) -> ("error out"=w991:errorcluster)  [unwired: 6 in, 6 out]
      }
      frame "Relay Pressure" {
        n566 = local read "Man Pres Control"() -> (w998:T17)
        n567 = Unbundle By Name(w998) -> ("Vial1"=w1008:bool, "Vial2"=w1007:bool, "Vial3"=w1006:bool, "Vial4"=w1005:bool, "Vent"=w1002:bool, "Pressure"=w1001:bool, "Pinch Valve"=w995:bool)
        n568 = Build Array(w1008, w1007, w1006, w1005, w1002, w1001) -> (w1004:bool[])
        n569 = Select(t=DAQ_Mngr."Pinch Valve Engage" ("DAQ Mngr Action"), s=w995, f=DAQ_Mngr."Pinch Valve Disengage" ("DAQ Mngr Action")) -> (s? t:f=w994:T38)
        n570 = call "DAQ Manager.vi"("DAQ Mngr Action"=w994, "error in (no error)"=w1000) -> ("error out"=w999:errorcluster)  [unwired: 7 in, 6 out]
        n571 = call "Denkovi Manager.vi"("Action"=Denkovi_Mngr."Set Pressure", "error in (no error)"=w999, "Relays In"=w1004) -> ("error out"=w1009:errorcluster)  [unwired: 6 in, 2 out]
      }
      frame "Relay Peristaltic" {
        n572 = local read "Man Peristaltic Ctrl"() -> (w1011:bool)
        n573 = Build Array(w1011) -> (w1013:bool[])
        n574 = call "Denkovi Manager.vi"("Action"=Denkovi_Mngr."Set Peristaltic", "error in (no error)"=w1015, "Relays In"=w1013) -> ("error out"=w1014:errorcluster)  [unwired: 6 in, 2 out]
      }
      frame "Pump Init" {
        w1021 = refnum<vi> refnum  # Slide
        n575 = control-ref of="Syringe Pump"() -> (w1024:refnum<vi>)
        n576 = property class="Clust (strict)"(reference=w1024) -> ("Controls[]"=w1023:refnum<vi>[])  [unwired: 1 in, 2 out]
        n577 = local read "Config"() -> (w1025:T1)
        n578 = Unbundle By Name(w1025) -> ("Syringe size"=w1017:u32)
        n579 = Index Array(array=w1023) -> (element=w1022:refnum<vi>)  [unwired: 1 in]
        n580 = To More Specific Class(target class=w1021, reference=w1022) -> (specific class reference=w1020:refnum<vi>)  [unwired: 1 in, 1 out]
        n581 = call "Tecan Mngr.vi"("Mngr Action"=Tricon_Mngr."Init Pump", "error in (no error)"=w1029) -> ("Raw Response"=w1019:string, "error out"=w1027:errorcluster)  [unwired: 8 in, 4 out]
        n582 = property class="Slide"(reference=w1020, "Scale.Minimum"=0.0 ("Scale.Range:Maximum"), "Scale.Maximum"=w1017) -> ()  [unwired: 1 in, 2 out]
        n583 = local write "Pump Response"(w1019) -> ()
        n584 = flat-sequence {
          tunnel: w1027 -> [w1036]
          tunnel: [w1036] -> w1026
          frame #0 {
            n585 = local read "Syringe Pump"() -> (w1035:T18)
            n586 = Bundle By Name(cluster=w1035, "Action"=enum32{"Withdraw", "Dispense", "Stop"}."Stop", "Syringe Pos"=u32 0, "Init"=FALSE) -> (w1033:T18)
            n587 = local write "Syringe Pump"(w1033) -> ()
          }
        }
      }
      frame "Pump Start" {
        n588 = local read "Syringe Pump"() -> (w1042:T18)
        n589 = call "Tecan Mngr.vi"("Mngr Action"=Tricon_Mngr."Start Pump", "Pump Data"=w1042, "error in (no error)"=w1044) -> ("Raw Response"=w1038:string, "Output Value"=w1041:dbl, "error out"=w1037:errorcluster)  [unwired: 7 in, 3 out]
        n590 = local write "Pump Response"(w1038) -> ()
        n591 = Bundle By Name(cluster=w1042, "Syringe Pos"=w1041, "Action"=enum32{"Withdraw", "Dispense", "Stop"}."Stop") -> (w1039:T18)
        n592 = local write "Syringe Pump"(w1039) -> ()
      }
      frame "Pump Start Abs" {
        n593 = local read "Syringe Pump"() -> (w1047:T18)
        n594 = call "Tecan Mngr.vi"("Mngr Action"=Tricon_Mngr."Start Pump", "Pump Data"=w1047, "error in (no error)"=w1053) -> ("Raw Response"=w1046:string, "Output Value"=w1048:dbl, "error out"=w1051:errorcluster)  [unwired: 7 in, 3 out]
        n595 = Bundle By Name(cluster=w1047, "Syringe Pos"=w1048, "Action"=enum32{"Withdraw", "Dispense", "Stop"}."Stop") -> (w1050:T18)
        n596 = local write "Pump Response"(w1046) -> ()
        n597 = local write "Syringe Pump"(w1050) -> ()
      }
      frame "Pump Set Valve" {
        n598 = local read "Syringe Pump"() -> (w1056:T18)
        n599 = call "Tecan Mngr.vi"("Mngr Action"=Tricon_Mngr."Set Valve", "Pump Data"=w1056, "error in (no error)"=w1059) -> ("Raw Response"=w1055:string, "error out"=w1057:errorcluster)  [unwired: 7 in, 4 out]
        n600 = local write "Pump Response"(w1055) -> ()
      }
      frame "Pump - Send Cmd" {
        n601 = local read "Pump Cmd"() -> (w1064:string)
        n602 = call "Tecan Mngr.vi"("Mngr Action"=Tricon_Mngr."Cmd", "Cmd"=w1064, "error in (no error)"=w1066) -> ("Raw Response"=w1063:string, "error out"=w1062:errorcluster)  [unwired: 7 in, 4 out]
        n603 = local write "Pump Response"(w1063) -> ()
        n604 = flat-sequence {
          tunnel: w1062 -> [w1069]
          tunnel: [w1069] -> w1061
          frame #0 {
            n605 = local write "Send Cmd"(FALSE ("Send Cmd")) -> ()
          }
        }
      }
      frame Default {
        n606 = disable-structure shown="Disabled" {
          disable-tunnel: w1071 -> [w1074 _]
          frame Disabled {
            n607 = Concatenate Strings("unkown queue msg:\n" ("string"), w1074) -> (w1073:string)
            n608 = One Button Dialog(message=w1073) -> ()  [unwired: 1 in, 1 out]
          }
          frame Enabled {
          }
        }
      }
      frame "Quit" {
        n609 = call "Zaber Manager.vi"("Action"=Mot_Stage_Mngr."Close", "error in (no error)"=w1076) -> ("error out"=w1075:errorcluster)  [unwired: 7 in, 6 out]
        n610 = call "Denkovi Manager.vi"("Action"=Denkovi_Mngr."Close", "error in (no error)"=w1076) -> ("error out"=w1078:errorcluster)  [unwired: 7 in, 2 out]
        n611 = call "DAQ Manager.vi"("DAQ Mngr Action"=DAQ_Mngr."Close", "error in (no error)"=w1076) -> ("error out"=w1079:errorcluster)  [unwired: 7 in, 6 out]
        n612 = call "Valco Valve Mngr.vi"("Mngr Action"=Valco_Valve_Mngr_Action."Close", "error in (no error)"=w1076) -> ("error out"=w1080:errorcluster)  [unwired: 9 in, 4 out]
        n613 = call "Tecan Mngr.vi"("Mngr Action"=Tricon_Mngr."Close", "error in (no error)"=w1076) -> ("error out"=w1087:errorcluster)  [unwired: 8 in, 5 out]
        n614 = Merge Errors(w1075, w1078, w1079, w1087, w1080) -> (w1081:errorcluster)
        n615 = call <userlib>:"MGI Is Runtime.vi"() -> ("Run Time System?"=w1085:bool)  [unwired: 7 in]
        n616 = case shown="False" w1085 {
          tunnel: w1081 -> [w1090 w1092]
          tunnel: [w1090 w1091] -> w1086
          frame False {
          }
          frame True {
            n617 = call <userlib>:"MGI Close Window.vi"("error in (no error)"=w1092) -> ("error out"=w1091:errorcluster)  [unwired: 10 in]
          }
        }
      }
    }
    n618 = call "Error Logger.vi"("Action"=T27."Update", "error in"=w579) -> ("error out"=w578:errorcluster)  [unwired: 8 in, 1 out]
  }
  n619 = while "NIDAQ" {
    tunnel: w8 -> [w1101]
    tunnel: w14 -> [w1097]
    tunnel: [w1094] -> w11
    stop <- w1100 stop-if-true
    n620 = Dequeue Element(queue=w1101) -> (queue out=w1093:refnum<queue>, element=w1098:string, error out=w1099:errorcluster)  [unwired: 2 in, 1 out]
    n621 = case shown="\"Quit\", Default" w1098 {
      tunnel: [TRUE _] -> w1100
      tunnel: w1099 -> [w1102 w1117]
      tunnel: [w1102 w1110] -> w1096
      tunnel: w1097 -> [_ _]
      tunnel: w1093 -> [_ w1107]
      frame "Quit", Default {
      }
      frame "Read Pressure" {
        n622 = call "DAQ Manager.vi"("DAQ Mngr Action"=DAQ_Mngr."Read Pressure", "error in (no error)"=w1117) -> ("error out"=w1114:errorcluster)  [unwired: 7 in, 6 out]
        n623 = local read "Fit Pnts"() -> (w1111:dbl)
        n624 = call "DAQ Manager.vi"("DAQ Mngr Action"=DAQ_Mngr."Analyze Pressure", "Value"=w1111, "error in (no error)"=w1114) -> ("Data Array"=w1104:T22[], "Plots"=w1113:T39[], "error out"=w1108:errorcluster)  [unwired: 6 in, 4 out]
        "Data Array" <- w1104
        n625 = local write "Pressure Level"(w1113) -> ()
        n626 = Enqueue Element(queue=w1107, element="Read Pressure", error in (no error)=w1108) -> (error out=w1106:errorcluster)  [unwired: 1 in, 2 out]
        n627 = call "Data Logger.vi"("Action"=enum16{"Init", "Save", "Close"}."Save", "error in"=w1106, "Data Array In"=w1104) -> ("error out"=w1110:errorcluster)  [unwired: 8 in]
        n628 = Wait (ms)(milliseconds to wait=u32 100) -> ()  [unwired: 1 out]
      }
    }
    n629 = call "Error Logger.vi"("Action"=T27."Update", "error in"=w1096) -> ("error out"=w1094:errorcluster)  [unwired: 8 in, 1 out]
  }
  n630 = Release Queue(queue=w21, error in (no error)=w30) -> ()  [unwired: 1 in, 3 out]
  n631 = Release Queue(queue=w8, error in (no error)=w11) -> ()  [unwired: 1 in, 3 out]
  n632 = Release Queue(queue=w26, error in (no error)=w35) -> ()  [unwired: 1 in, 3 out]
  "Version" <- "1.2.2" ("Version")
